vi "891 Software.vi"() -> ()   [LabVIEW 2020]
doc: "This Continuous Measurement sample project is based on the Queued Message Handler template.\n\nThe Event Handling Loop generates messages based on user interface actions.\n\nThe Message Handling Loop processes messages generated by the Event Handling Loop, or by other messages. There are also Acquisition and Logging message handling loop subVIs, and a chart updating loop."
uses:
  2840 Software/controls/Instrument Refs.ctl
  Settings/Settings.ctl
  controls/UI Data.ctl
  controls/UI State.ctl
  controls/UI Sweep.ctl
  support/Message Queue/Enqueue Message (Single).vi
  support/Message Queue/Enqueue Message (Array).vi
  <vilib>/Utility/error.llb/Error Cluster From Error Code.vi
  <vilib>/regexp/Match Regular Expression.xnode
  <vilib>/ErrorRing/Error Ring.xnode
  Acquisition/Acquisition.lvlib
  Logging/Logging.lvlib
  Settings/Settings.lvlib
  support/User Event - Stop/User Event - Stop.lvlib
  support/Message Queue/Message Queue.lvlib
  891 software library/Copy of Copy of BK Precision 891.lvlib
  Settings/Settings Dialog.vi
panel:
  in  "Disconnect":bool
  out "Enable Sweep New Value":bool
  out "NewVal":enum32{"BIN", "SWEEP"}(ring)
  out "Tab Ref":refnum<vi>
  out "OldVal":dbl
  out "CtlRef":refnum<vi>
  out "New High Limit Val":dbl
  out "High Limit Ref":refnum<vi>
  out "Low Limit Ref":refnum<vi>
  out "New Low Limit Val":dbl
  out "BIN REF":refnum<vi>
  out "New BIN State":bool
  in  "BIN Read In":T1
  in  "?":T2
  out "Function":string
  out "Secondary":string
  out "Primary":string
  out "Color Box":u32(colorbox)=11347
  in  "Frequency":dbl=1000.0 format="%#_4p"
  in  "Level":u8(ring) items=["0.5Vrms", "1Vrms"]
  in  "Range":u16(ring)=1 items=["Hold", "Auto"]
  in  "Speed":u16(ring)=1 items=["Slow"=1, "Fast"=2]
  in  "Function":u16(ring) items=["Cs-Q", "Cs-D", "Cs-R", "Cp-Q", "Cp-D", "Cp-R", "Cp-G", "Ls-Q", "Ls-D", "Ls-R", "Lp-Q", "Lp-D", "Lp-R", "Lp-G", "Z-th", "Y-th", "R-X", "G-B", "DCR"]
  in  "Tab Control":enum32{"BIN", "SWEEP"}(tab)
  in  "High Limit":T3={"BIN 1"=1.0, "BIN 2"=1.0, "BIN 3"=1.0, "BIN 4"=1.0, "BIN 5"=1.0, "BIN 6"=1.0, "BIN 7"=1.0, "BIN 8"=1.0, "BIN 9"=1.0, "SEC"=1.0} {"SEC" min=1.0 step=100.0 format="%#_6p"; "BIN 9" min=1.0 step=100.0 format="%#_6p"; "BIN 8" min=1.0 step=100.0 format="%#_6p"; "BIN 7" min=1.0 step=100.0 format="%#_6p"; "BIN 6" min=1.0 step=100.0 format="%#_6p"; "BIN 5" min=1.0 step=100.0 format="%#_6p"; "BIN 4" min=1.0 step=100.0 format="%#_6p"; "BIN 3" min=1.0 step=100.0 format="%#_6p"; "BIN 2" min=1.0 step=100.0 format="%#_6p"; "BIN 1" min=1.0 step=100.0 format="%#_6p"}
  in  "Low Limit":T3 {"SEC" step=100.0 format="%#_6p"; "BIN 9" step=100.0 format="%#_6p"; "BIN 8" step=100.0 format="%#_6p"; "BIN 7" step=100.0 format="%#_6p"; "BIN 6" step=100.0 format="%#_6p"; "BIN 5" step=100.0 format="%#_6p"; "BIN 4" step=100.0 format="%#_6p"; "BIN 3" step=100.0 format="%#_6p"; "BIN 2" step=100.0 format="%#_6p"; "BIN 1" step=100.0 format="%#_6p"}
  in  "BIN State Read":bool
  in  "Clear Count":bool=TRUE
  in  "Comparator Swap":bool
  in  "Trigger":bool=TRUE
  in  "Count State":bool
  in  "Beeper Mode":u16(ring) items=["Off", "Beep when Pass", "Beep when Failed"]
  in  "Comparator Mode":u16(ring) items=["Tolerance", "Absolute"]
  in  "Bin Display Mode":u16(ring) items=["BIN", "Table", "Histogram"]
  in  "Nominal Value (0.0)":dbl step=100.0
  in  "BIN No.":T4
  out "BIN 1":bool
  out "BIN 2":bool
  out "BIN 3":bool
  out "BIN 4":bool
  out "BIN 5":bool
  out "BIN 6":bool
  out "BIN 7":bool
  out "BIN 8":bool
  out "BIN 9":bool
  out "BIN 10":bool
  out "BIN Result":i32[](array[numeric]) format="%.0p"
  out "Nominal":string
  out "Low Limit Read":dbl[](array[numeric]) format="%#_6p"
  out "High Limit Read":dbl[](array[numeric]) format="%#_6p"
  in  "Sweep Function":u16(ring) items=["Cs-Q", "Cs-D", "Cs-R", "Cp-Q", "Cp-D", "Cp-R", "Cp-G", "Ls-Q", "Ls-D", "Ls-R", "Lp-Q", "Lp-D", "Lp-R", "Lp-G", "Z-th", "Y-th", "R-X", "G-B", "DCR"]
  out "XY Graph":cluster{dbl[], dbl[]}(graph)
  in  "Interpolation":u16(ring) items=["Disable", "Enable"]
  in  "Sweep Display Mode":u16(ring) items=["Graph", "Table"]
  in  "Autoscale Limit":bool=TRUE
  in  "Sweep Low Limit":dbl format="%#.3f"
  in  "Sweep High Limit":dbl format="%#.3f"
  in  "Start Frequency":dbl=20.0 min=20.0 max=300000.0 format="%.1f"
  in  "Stop Frequency":dbl=1000.0 min=20.0 max=300000.0 format="%.1f"
  in  "Sweep Points":i32(ring) items=["300 ", "150", "60", "30"]
  in  "Autoscale Frequency":bool=TRUE
  in  "Sweep Parameter":u16(ring) items=["Primary", "Secondary"]
  in  "Sweep Mode":u16(ring) items=["Linear", "Logarithmic"]
  in  "Enable Sweep":bool
  in  "Log File Path":path
  in  "Connect":bool=TRUE
  in  "Reset (True)":bool=TRUE
  in  "Select LCR":refnum<visa-resource-name>="COM12"
  in  "Settings":bool
  in  "Start":bool
  in  "Stop":bool
  in  "Disconnect":bool
  out "FW Ver.":string="/ 1.68 / 4.02B\r\n"
  out "SN":string="BK001, 3."
  out "Model":string="891"
  out "IDN":string="B&K Precision ,891,BK001, 3.02/ 1.68 / 4.02B\r\n"
  out "Status":string="Exit"
  # "Measurement"
  # "Signal Configuration"
  # "1"
  # "2"
  # "3"
  # "4"
  # "5"
  # "6"
  # "7"
  # "8"
  # "9"
  # "SEC"
  # "OUT"
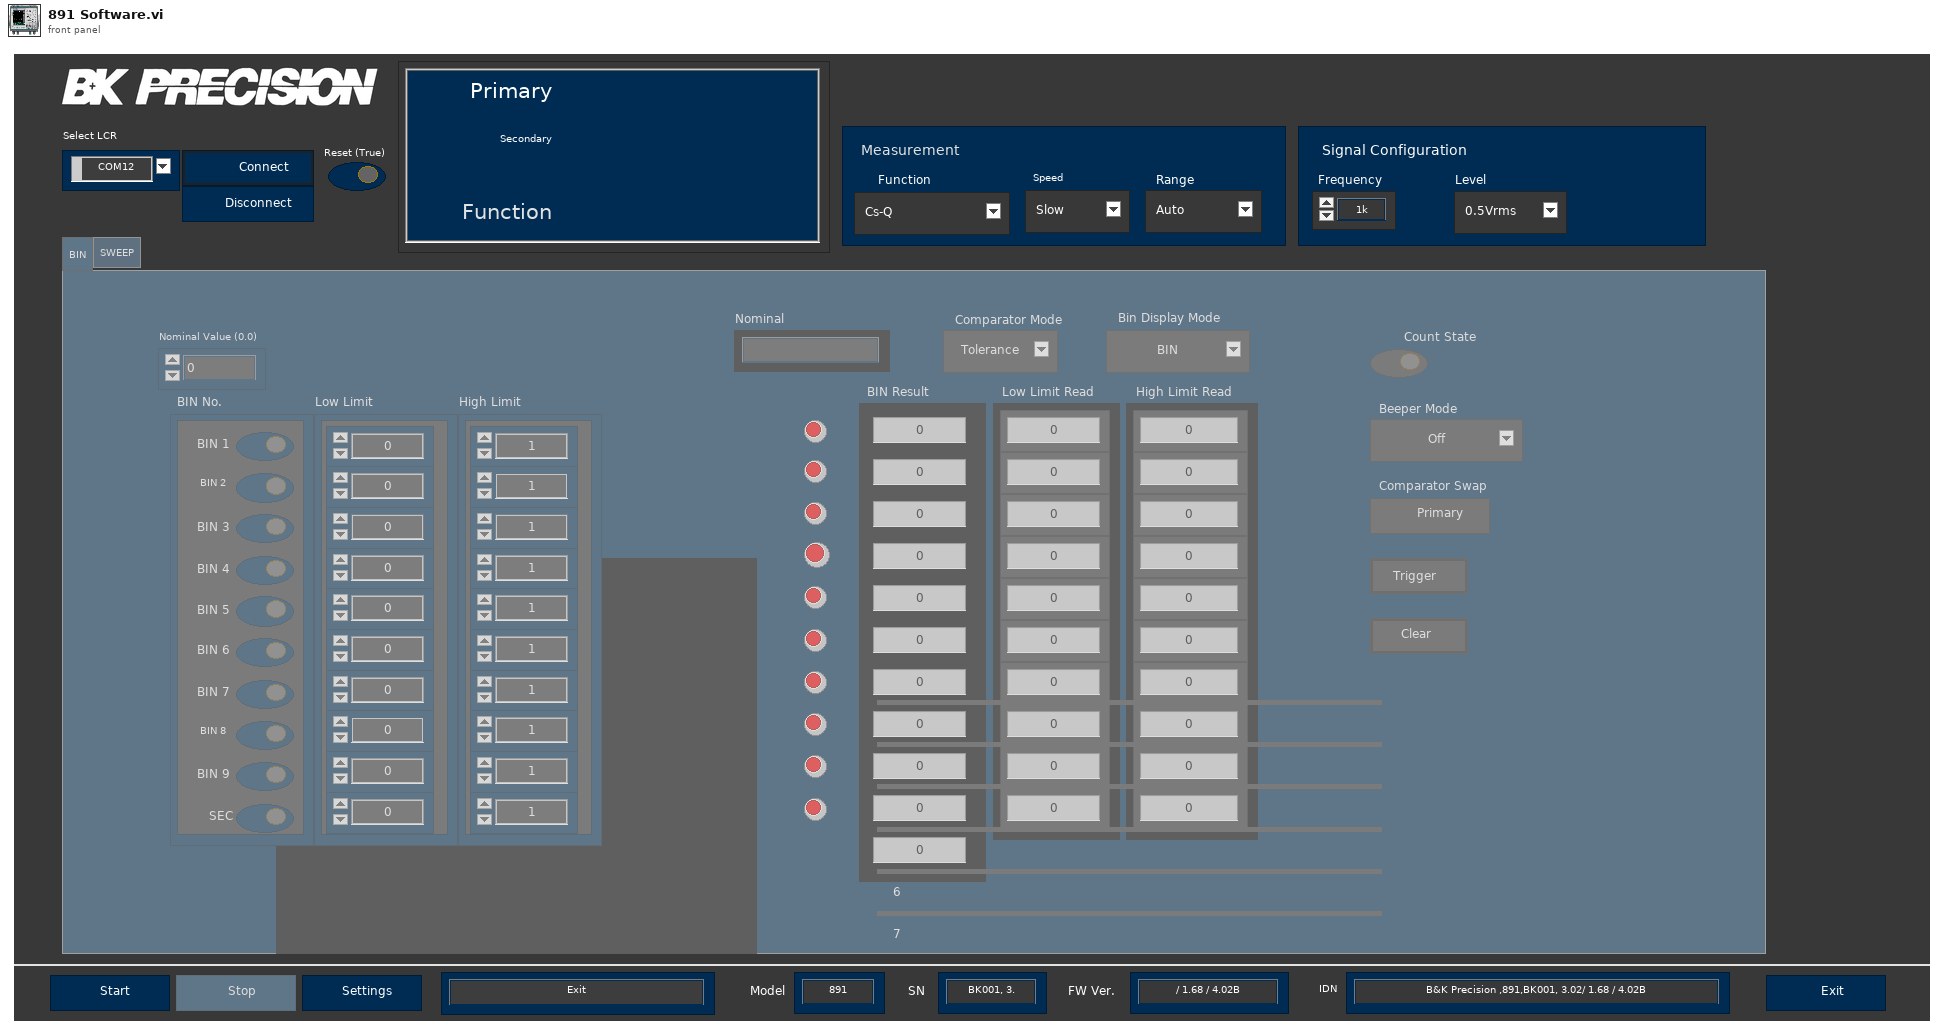
[diagram p1: front panel]
types:
  T1 = cluster{"Low Limit Read":dbl[], "High Limit Read":dbl[], "BIN Count Array":i32[], "Nominal":string}
  T2 = typedef "Instrument Refs.ctl" = cluster{"Function":refnum<vi>, "BIN 1":refnum<vi>, "BIN 2":refnum<vi>, "BIN 3":refnum<vi>, "BIN 4":refnum<vi>, "BIN 5":refnum<vi>, "BIN 6":refnum<vi>, "BIN 7":refnum<vi>, "BIN 8":refnum<vi>, "BIN 9":refnum<vi>, "BIN 10":refnum<vi>}
  T3 = cluster{"BIN 1":dbl, "BIN 2":dbl, "BIN 3":dbl, "BIN 4":dbl, "BIN 5":dbl, "BIN 6":dbl, "BIN 7":dbl, "BIN 8":dbl, "BIN 9":dbl, "SEC":dbl}
  T4 = cluster{"BIN 1":bool, "BIN 2":bool, "BIN 3":bool, "BIN 4":bool, "BIN 5":bool, "BIN 6":bool, "BIN 7":bool, "BIN 8":bool, "BIN 9":bool, "SEC":bool}
  T5 = typedef "UI Sweep.ctl" = cluster{"Function Ref":refnum<vi>, "Speed Ref":refnum<vi>, "Range Ref":refnum<vi>, "Comparator Ref":refnum<vi>, "BIN Display Ref":refnum<vi>, "Enable Count Ref":refnum<vi>, "Beeper Ref":refnum<vi>, "BIN NO. Ref":refnum<vi>, "Low Limit Ref":refnum<vi>, "High Limit Ref":refnum<vi>, "Nominal Value Ref":refnum<vi>, "Enable Sweep":refnum<vi>, "Sweep Mode Ref":refnum<vi>, "Sweep Display Mode Ref":refnum<vi>, "Sweep Parameter Ref":refnum<vi>, "Interporlation Ref":refnum<vi>, "Sweep Step Ref":refnum<vi>, "Autoscale Sweep":refnum<vi>, "Start Freq Ref":refnum<vi>, "Stop Freq Ref":refnum<vi>, "Autoscale Frequency":refnum<vi>, "Sweep Low Limit Ref":refnum<vi>, "Sweep High Limit Ref":refnum<vi>, "Freq Ref":refnum<vi>, "Level Ref":refnum<vi>, "TabCtl Refnum":refnum<vi>}
  T6 = typedef "UI State.ctl" = enum16{"Idle", "Acquiring and Logging", "Waiting for Exit", "Waiting for Exit (Acq Stopped)", "Waiting for Exit (Log Stopped)", "Waiting for Stop", "Waiting for Stop (Acq Stopped)", "Waiting for Stop (Log Stopped)", "Waiting for Sweep(Sweep Complete)"}
  T7 = typedef "UI Data.ctl" = cluster{"Start Ref":refnum<vi>, "Stop Ref":refnum<vi>, "Settings Ref":refnum<vi>, "Exit Ref":refnum<vi>, "Status Ref":refnum<vi>, "Function Ref":refnum<vi>, "Range Ref":refnum<vi>, "Speed Ref":refnum<vi>, "Level Ref":refnum<vi>, "Freq Refnum":refnum<vi>, "Sweep ":refnum<vi>, "Autoscale Sweep":refnum<vi>, "Autoscale Frequency":refnum<vi>, "TabCtl Refnum":refnum<vi>}
  T8 = typedef "Settings.lvlib/Settings.ctl" = cluster{"VISA resource name":refnum<visa-resource-name>, "Logging Configuration":cluster{"Byte Stream File Refnum":refnum<file>, "File Path":path, "String":string}, "Comparator Mode":u16, "BIN State":bool, "Start Ref":refnum<vi>, "Stop Ref":refnum<vi>}
  T9 = typedef "Message Queue.lvlib/All Message Queues.ctl" = cluster{"UI":refnum<queue>, "Acquisition":refnum<queue>, "Logging":refnum<queue>}
  T10 = enum8{"Enabled", "Disabled", "Disabled and Grayed Out"}
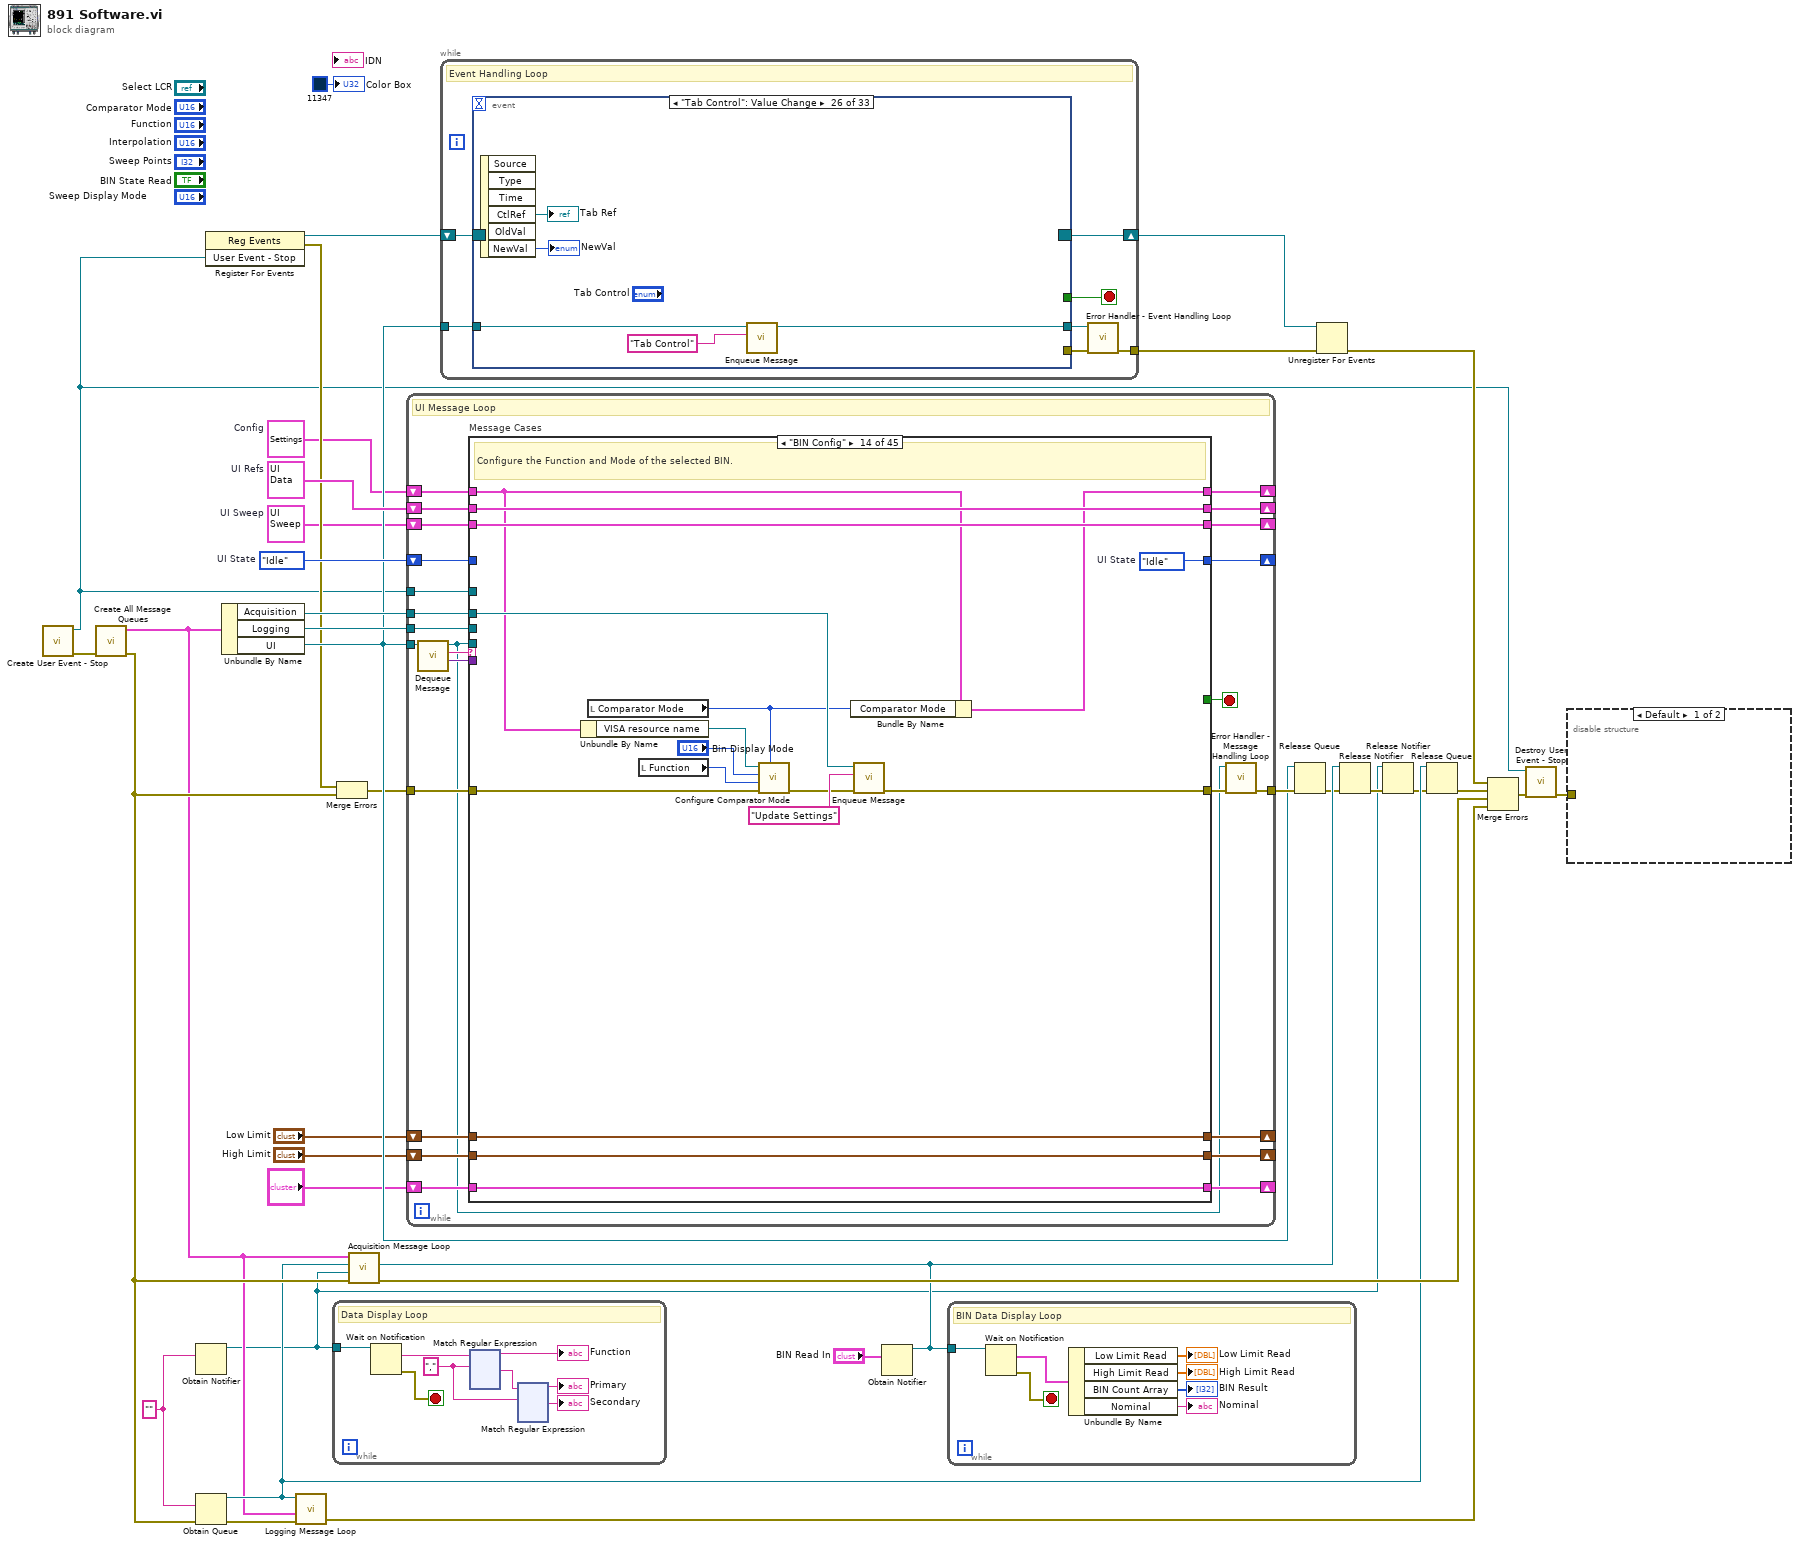
[diagram p0: block diagram]
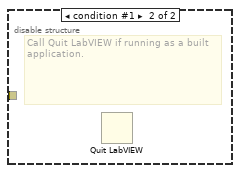
[diagram p2: hidden frame]
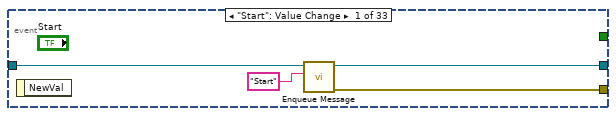
[diagram p3: hidden frame]
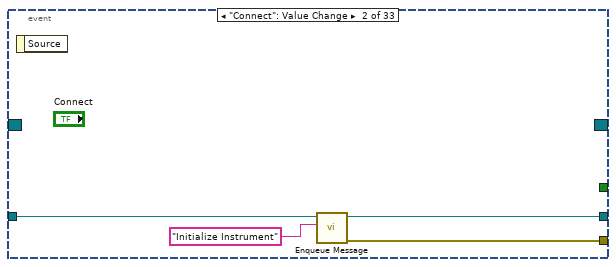
[diagram p4: hidden frame]
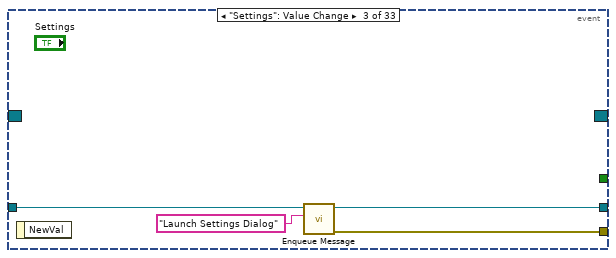
[diagram p5: hidden frame]
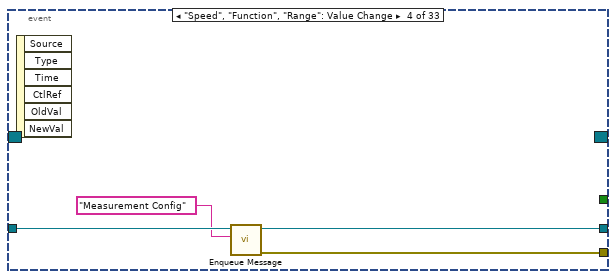
[diagram p6: hidden frame]
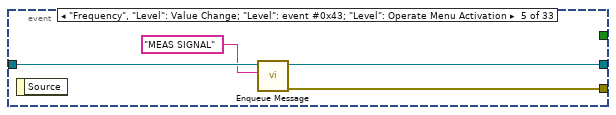
[diagram p7: hidden frame]
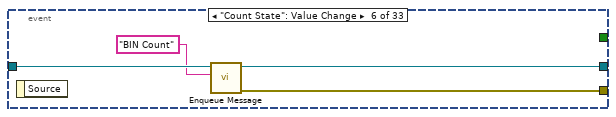
[diagram p8: hidden frame]
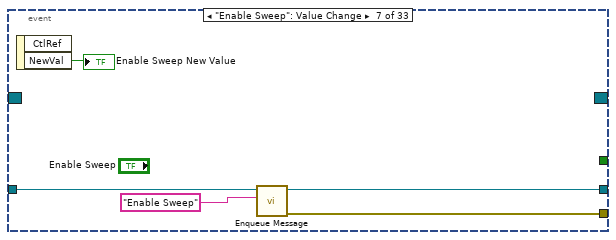
[diagram p9: hidden frame]
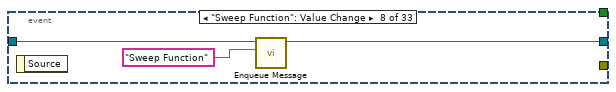
[diagram p10: hidden frame]
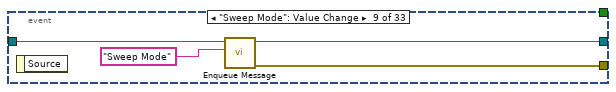
[diagram p11: hidden frame]
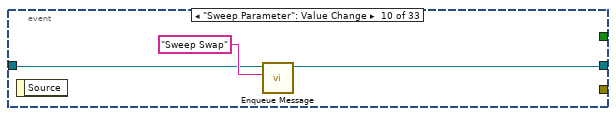
[diagram p12: hidden frame]
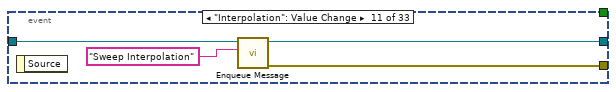
[diagram p13: hidden frame]
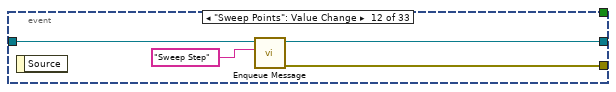
[diagram p14: hidden frame]
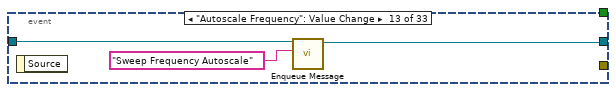
[diagram p15: hidden frame]
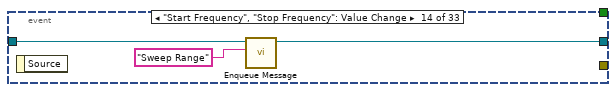
[diagram p16: hidden frame]
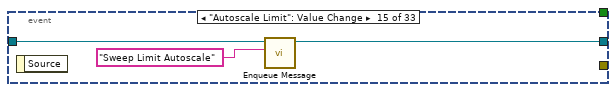
[diagram p17: hidden frame]
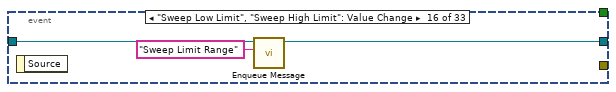
[diagram p18: hidden frame]
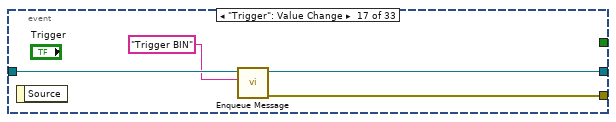
[diagram p19: hidden frame]
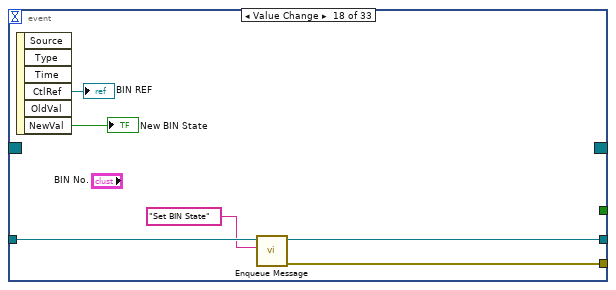
[diagram p20: hidden frame]
diagram:
  w18 = T5 {"Function Ref"=refnum, "Speed Ref"=refnum, "Range Ref"=refnum, "Comparator Ref"=refnum, "BIN Display Ref"=refnum, "Enable Count Ref"=refnum, "Beeper Ref"=refnum, "BIN NO. Ref"=refnum, "Low Limit Ref"=refnum, "High Limit Ref"=refnum, "Nominal Value Ref"=refnum, "Enable Sweep"=refnum, "Sweep Mode Ref"=refnum, "Sweep Display Mode Ref"=refnum, "Sweep Parameter Ref"=refnum, "Interporlation Ref"=refnum, "Sweep Step Ref"=refnum, "Autoscale Sweep"=refnum, "Start Freq Ref"=refnum, "Stop Freq Ref"=refnum, "Autoscale Frequency"=refnum, "Sweep Low Limit Ref"=refnum, "Sweep High Limit Ref"=refnum, "Freq Ref"=refnum, "Level Ref"=refnum, "TabCtl Refnum"=refnum}  # UI Sweep
  w20 = ""
  w27 = UI_State."Idle"  # UI State
  w30 = T7 {"Start Ref"=refnum, "Stop Ref"=refnum, "Settings Ref"=refnum, "Exit Ref"=refnum, "Status Ref"=refnum, "Function Ref"=refnum, "Range Ref"=refnum, "Speed Ref"=refnum, "Level Ref"=refnum, "Freq Refnum"=refnum, "Sweep "=refnum, "Autoscale Sweep"=refnum, "Autoscale Frequency"=refnum, "TabCtl Refnum"=refnum}  # UI Refs
  w17 = T8 {"VISA resource name"="COM1", "Logging Configuration"={"Byte Stream File Refnum"=refnum, "File Path"=path "", "String"=""}, "Comparator Mode"=1, "BIN State"=FALSE, "Start Ref"=refnum, "Stop Ref"=refnum}  # Config
  n1 = call "Create User Event - Stop.vi"() -> ("error out"=w33:errorcluster, "User Event - Stop"=w4:refnum<user-event>)  [unwired: 10 in]
  n2 = call "Create All Message Queues.vi"("error in (no error)"=w33) -> ("error out"=w15:errorcluster, "Message Queues out"=w9:T9)  [unwired: 9 in]
  n3 = Obtain Notifier(notification data type=w20) -> (notifier out=w5:refnum<notifier>)  [unwired: 3 in, 2 out]
  n4 = Obtain Queue(element data type=w20, error in (no error)=w15) -> (queue out=w10:refnum<queue>, error out=w16:errorcluster)  [unwired: 3 in, 1 out]
  n5 = register-events(w4) -> (reference out=w23:refnum<event-registration>, error out=w21:errorcluster)  [unwired: 2 in]
  n6 = Unbundle By Name(w9) -> ("Acquisition"=w29:refnum<queue>, "Logging"=w28:refnum<queue>, "UI"=w25:refnum<queue>)
  n7 = call "Logging Message Loop.vi"("error in (no error)"=w16, "Message Queues"=w9, "Data Queue"=w10) -> ("error out"=w32:errorcluster)  [unwired: 8 in]
  n8 = while "Data Display Loop" {
    tunnel: w5 -> [w44]
    stop <- w43 stop-if-true
    w39 = "," ("regular expression")
    # "Data Display Loop"
    n9 = Wait on Notification(notifier=w44) -> (notification=w40:string, error out=w43:errorcluster)  [unwired: 3 in, 2 out]
    n10 = xnode "Match Regular Expression"("input string"=w40, "regular expression"=w39) -> ("before match"=→"Function":string, "after match"=w38:string)  [unwired: 4 in, 3 out]
    n11 = xnode "Match Regular Expression"("input string"=w38, "regular expression"=w39) -> ("before match"=→"Primary":string, "after match"=→"Secondary":string)  [unwired: 4 in, 3 out]
  }
  n12 = Merge Errors(w21, w15) -> (w22:errorcluster)
  n13 = while {
    tunnel: w25 -> [w293]
    tunnel: w4 -> [w296]
    shift-right: [w292] -> _
    shift-left: w17 -> [w278]
    shift-right: [w290] -> _
    shift-left: w30 -> [w291]
    tunnel: w29 -> [w289]
    tunnel: w28 -> [w288]
    shift-right: [w284] -> _
    shift-left: w27 -> [w285]
    tunnel: w22 -> [w283]
    tunnel: [w287] -> w36
    shift-right: [w281] -> _
    shift-left: w18 -> [w282]
    shift-right: [w279] -> _
    shift-left: "?" -> [w280]
    shift-right: [w274] -> _
    shift-left: "High Limit" -> [w277]
    shift-right: [w275] -> _
    shift-left: "Low Limit" -> [w276]
    stop <- w297 stop-if-true
    # "UI Message Loop"
    n14 = call "Dequeue Message.vi"("Message Queue"=w293) -> ("Message Data"=w294:variant, "Message"=w295:string, "dup Message Queue"=w273:refnum<queue>)  [unwired: 7 in, 1 out]
    n15 = case "Message Cases" shown="\"BIN Config\"" w295 {
      selector: w295 -> [_ _ _ _ _ _ _ _ _ _ _ _ _ _ _ _ _ _ _ _ _ _ _ _ _ _ _ _ _ _ _ _ _ _ _ _ _ _ _ _ _ _ _ _ w1651]
      tunnel: w273 -> [w306 _ _ w389 _ w431 _ _ _ _ _ _ _ _ _ _ _ _ _ w1051 _ _ _ _ _ _ _ _ _ _ w1296 w1333 w1380 _ w1428 w1465 w1496 _ _ w1543 w1579 _ _ _ _]
      tunnel: w283 -> [w309 w322 w376 w412 w425 w433 w461 w491 w504 w526 w665 w812 w945 w970 w985 w995 w1019 w1029 w1047 w1058 w1147 w1163 w1175 w1195 w1210 w1224 w1245 w1252 w1268 w1282 w1298 w1363 w1398 w1418 w1429 w1466 w1498 w1521 w1529 w1542 w1570 w1597 w1623 w1641 _]
      tunnel: [w313 w322 w376 w390 w426 w450 w460 w490 w503 w524 w662 w809 w944 w966 w984 w990 w1016 w1025 w1037 w1061 w1146 w1162 w1173 w1194 w1209 w1223 w1245 w1251 w1267 w1281 w1294 w1336 w1382 w1403 w1426 w1463 w1492 w1522 w1527 w1541 w1571 w1594 w1620 w1641 w1650] -> w286
      tunnel: [_ _ _ _ _ _ _ _ _ _ _ _ _ _ _ _ _ _ _ _ _ _ _ _ _ _ _ _ _ _ _ _ _ _ _ _ _ _ _ _ _ _ TRUE _ _] -> w297
      tunnel: w294 -> [_ _ _ _ w424 _ _ _ _ _ _ _ _ _ _ _ _ _ _ _ _ _ _ _ _ _ _ _ _ _ _ _ _ _ _ _ _ _ w1532 _ _ w1602 w1632 _ _]
      tunnel: w296 -> [_ _ _ _ _ _ _ _ _ _ _ _ _ _ _ _ _ _ _ _ _ _ _ _ _ _ _ _ _ _ _ _ _ _ _ _ _ _ _ _ _ _ w1628 _ _]
      tunnel: [w302 w338 w375 w397 w416 w448 w457 w486 w499 w523 w664 w811 w940 w964 w980 w998 w1014 w1031 w1042 w1059 w1143 w1159 w1176 w1193 w1207 w1222 w1236 w1250 w1270 w1278 w1292 w1356 w1378 w1401 w1423 w1458 w1491 w1512 w1525 w1537 w1573 w1588 w1626 w1639 w1647] -> w292
      tunnel: w291 -> [w310 w348 w380 w403 w420 w454 w466 w496 w508 w533 w669 w816 w950 w977 w988 w1002 w1022 w1035 w1049 w1062 w1155 w1170 w1183 w1198 w1217 w1230 w1244 w1258 w1274 w1289 w1301 w1360 w1396 w1417 w1431 w1457 w1494 w1520 w1534 w1545 w1583 w1605 w1635 w1644 w1653]
      tunnel: [w310 w346 w380 w403 w420 w454 w466 w496 w508 w533 w669 w816 w950 w977 w988 w1002 w1022 w1035 w1049 w1062 w1155 w1170 w1183 w1198 w1217 w1230 w1244 w1258 w1274 w1289 w1301 w1360 w1396 w1417 w1431 w1457 w1494 w1520 w1534 w1545 w1583 w1605 w1635 w1644 w1653] -> w290
      tunnel: w289 -> [_ _ _ _ _ w451 _ _ _ _ _ _ _ w968 _ w989 _ w1027 w1036 w1052 _ _ _ _ _ _ _ _ _ _ _ w1337 _ _ _ _ _ w1519 _ _ w1581 w1585 w1624 _ _]
      tunnel: w288 -> [_ _ _ _ _ _ _ _ _ _ _ _ _ _ _ _ _ _ _ _ _ _ _ _ _ _ _ _ _ _ _ _ w1386 w1407 _ _ _ w1518 _ _ w1576 w1586 w1625 _ _]
      tunnel: w285 -> [_ _ _ w413 w419 w453 w455 w494 w502 w531 w645 w796 w943 _ w982 w1000 w1017 w1033 w1045 w1055 w1145 w1167 w1181 w1191 w1205 w1227 w1241 w1255 w1272 w1279 _ w1339 _ w1405 w1430 w1467 w1493 w1517 w1531 w1544 w1580 _ _ w1643 w1652]
      tunnel: [UI_State."Idle" ("UI State") UI_State."Idle" ("UI State") w379 w413 w419 w453 w455 w494 w502 w531 w645 w796 w943 w976 w982 w1000 w1017 w1033 w1045 w1055 w1145 w1167 w1181 w1191 w1205 w1227 w1241 w1255 w1272 w1279 w1300 w1339 UI_State."Acquiring and Logging" ("UI State") w1406 w1427 w1464 w1493 w1517 w1531 w1540 w1580 UI_State."Idle" ("UI State") UI_State."Idle" ("UI State") w1643 w1652] -> w284
      tunnel: [w300 w336 w377 w398 w418 w452 w465 w495 w501 w532 w668 w815 w949 w975 w987 w1001 w1021 w1034 w1048 w1056 w1144 w1169 w1182 w1187 w1216 w1229 w1243 w1257 w1273 w1280 w1299 w1355 w1384 w1404 w1425 w1462 w1490 w1516 w1528 w1539 w1582 w1592 w1616 w1642 w1649] -> w281
      tunnel: w282 -> [w301 w336 w378 w398 w418 w452 w465 w495 w501 w532 w668 w815 w949 w975 w987 w1001 w1021 w1034 w1048 w1056 w1144 w1169 w1182 w1187 w1216 w1229 w1243 w1257 w1273 w1280 w1299 w1355 w1384 w1404 w1425 w1462 w1490 w1516 w1528 w1539 w1582 w1592 w1616 w1642 w1649]
      tunnel: w280 -> [w304 w334 w353 w388 w417 w434 w464 w487 w500 w530 w667 w814 w948 w974 w981 w999 w1015 w1032 w1043 w1060 w1154 w1168 w1180 w1197 w1215 w1228 w1242 w1256 w1271 w1288 w1293 w1357 w1379 w1402 w1424 w1461 w1489 w1507 w1526 w1538 w1574 w1598 w1627 w1640 w1648]
      tunnel: [w304 w333 w353 w388 w417 w434 w464 w487 w500 w530 w667 w814 w948 w974 w981 w999 w1015 w1032 w1043 w1060 w1154 w1168 w1180 w1197 w1215 w1228 w1242 w1256 w1271 w1288 w1293 w1357 w1379 w1402 w1424 w1461 w1489 w1507 w1526 w1538 w1574 w1598 w1627 w1640 w1648] -> w279
      tunnel: w278 -> [w303 w321 w375 w387 w416 w448 w457 w486 w499 w523 w664 w811 w940 w965 w980 w998 w1014 w1031 w1042 w1059 w1143 w1159 w1176 w1193 w1207 w1222 w1236 w1250 w1270 w1278 w1292 w1356 w1378 w1401 w1423 w1458 w1488 w1506 w1525 w1537 w1573 w1588 w1626 w1639 w1647]
      tunnel: w277 -> [w298 w317 w349 w382 w414 w427 w462 w484 w497 w509 w648 w793 w946 w961 w978 w992 w1012 w1023 w1040 w1053 w1136 w1156 w1171 w1188 w1203 w1218 w1233 w1246 w1261 w1275 w1290 w1329 w1376 w1399 w1421 w1459 w1486 w1504 w1523 w1535 w1567 w1590 w1614 w1637 w1645]
      tunnel: w276 -> [w299 w318 w350 w383 w415 w428 w463 w485 w498 w510 w647 w794 w947 w962 w979 w993 w1013 w1024 w1041 w1054 w1137 w1157 w1172 w1189 w1204 w1219 w1234 w1247 w1262 w1276 w1291 w1330 w1377 w1400 w1422 w1460 w1487 w1505 w1524 w1536 w1568 w1591 w1615 w1638 w1646]
      tunnel: [w299 w318 w350 w383 w415 w428 w463 w485 w498 w510 w646 w794 w947 w962 w979 w993 w1013 w1024 w1041 w1054 w1137 w1157 w1172 w1189 w1204 w1219 w1234 w1247 w1262 w1276 w1291 w1330 w1377 w1400 w1422 w1460 w1487 w1505 w1524 w1536 w1568 w1591 w1615 w1638 w1646] -> w275
      tunnel: [w298 w317 w349 w382 w414 w427 w462 w484 w497 w509 w648 w792 w946 w961 w978 w992 w1012 w1023 w1040 w1053 w1136 w1156 w1171 w1188 w1203 w1218 w1233 w1246 w1261 w1275 w1290 w1329 w1376 w1399 w1421 w1459 w1486 w1504 w1523 w1535 w1567 w1590 w1614 w1637 w1645] -> w274
      frame "Initialize" {
        # "Initialize - Get configuration settings, then message the UI to initialize, and broadcast the settings to the other message loops."
        n16 = call-poly "Enqueue Message.vi"("error in (no error)"=w309, "Message Array"=string[] ["Init UI Refs", "Set Controls Ref", "Broadcast Settings"], "Message Queue"=w306) -> ("error out"=w314:errorcluster, "dup Message Queue"=w305:refnum<queue>)  [unwired: 7 in]
        n17 = call-poly "Enqueue Message.vi"("error in (no error)"=w314, "Message Data"="Ready..." ("Ready..."), "Message"="Update Status", "Message Queue"=w305) -> ("error out"=w313:errorcluster)  [unwired: 6 in, 1 out]
        n18 = call "Load Settings from XML.vi"("Settings in"=w303) -> ("Settings out"=w302:T8)  [unwired: 9 in, 1 out]
        n19 = call "Load Default UI Settings.vi"("UI Sweep"=w301) -> ("UI Sweep OUT"=w300:T5)  [unwired: 9 in, 1 out]
      }
      frame "Init UI Refs" {
        w319 = T10."Disabled and Grayed Out" ("Disabled")
        w320 = T10."Disabled and Grayed Out" ("Disabled")
        # "Init UI Refs - Store control references for UI controls.  Also enable/disable controls appropriately."
        n20 = control-ref of="BIN 1"() -> (w327:refnum<vi>)
        n21 = control-ref of="BIN 2"() -> (w328:refnum<vi>)
        n22 = control-ref of="BIN 3"() -> (w329:refnum<vi>)
        n23 = control-ref of="BIN 4"() -> (w330:refnum<vi>)
        n24 = control-ref of="BIN 5"() -> (w331:refnum<vi>)
        n25 = control-ref of="BIN 6"() -> (w332:refnum<vi>)
        n26 = control-ref of="BIN 7"() -> (w326:refnum<vi>)
        n27 = control-ref of="BIN 8"() -> (w325:refnum<vi>)
        n28 = control-ref of="BIN 9"() -> (w324:refnum<vi>)
        n29 = control-ref of="BIN 10"() -> (w323:refnum<vi>)
        n30 = control-ref of="Start"() -> (w316:refnum<vi>)
        n31 = control-ref of="Stop"() -> (w315:refnum<vi>)
        n32 = control-ref of="Settings"() -> (w341:refnum<vi>)
        n33 = control-ref of="Disconnect"() -> (w340:refnum<vi>)
        n34 = control-ref of="Tab Control"() -> (w335:refnum<vi>)
        n35 = property on="Start Frequency" class="DigNum (strict)"("DisabledEnum"=w320) -> ()  [unwired: 2 in, 2 out]
        n36 = property on="Stop Frequency" class="DigNum (strict)"("DisabledEnum"=w320) -> ()  [unwired: 2 in, 2 out]
        n37 = control-ref of="Status"() -> (w347:refnum<vi>)
        n38 = Build Array(w316, w341, w340) -> (w344:refnum<vi>[])
        n39 = Bundle By Name(cluster=w334, "BIN 1"=w327, "BIN 2"=w328, "BIN 3"=w329, "BIN 4"=w330, "BIN 5"=w331, "BIN 6"=w332, "BIN 7"=w326, "BIN 8"=w325, "BIN 9"=w324, "BIN 10"=w323) -> (w333:T2)
        n40 = call "Set Enable State on Multiple Controls.vi"("Enable?"=TRUE, "Controls"=w344) -> ()  [unwired: 10 in]
        n41 = Bundle By Name(cluster=w348, "Start Ref"=w316, "Stop Ref"=w315, "Settings Ref"=w341, "Exit Ref"=w340, "Status Ref"=w347, "TabCtl Refnum"=w335) -> (w346:T7)
        n42 = property on="Sweep Low Limit" class="DigNum (strict)"("DisabledEnum"=w319) -> ()  [unwired: 2 in, 2 out]
        n43 = property on="Sweep High Limit" class="DigNum (strict)"("DisabledEnum"=w319) -> ()  [unwired: 2 in, 2 out]
        n44 = Bundle By Name(cluster=w321, "Logging Configuration.File Path"="Log File Path") -> (w338:T8)
        n45 = Build Array(w315, w335) -> (w343:refnum<vi>[])
        n46 = call "Set Enable State on Multiple Controls.vi"("Enable?"=FALSE, "Controls"=w343) -> ()  [unwired: 10 in]
      }
      frame "Set Controls Ref" {
        w379 = UI_State."Idle"  # UI State
        # "BIN Refs"
        # "Sweep Config"
        # "Signal Config Ref"
        # "Measurement Ref"
        n47 = control-ref of="Count State"() -> (w370:refnum<vi>)
        n48 = control-ref of="Enable Sweep"() -> (w369:refnum<vi>)
        n49 = control-ref of="Autoscale Limit"() -> (w360:refnum<vi>)
        n50 = control-ref of="Autoscale Frequency"() -> (w357:refnum<vi>)
        n51 = control-ref of="BIN No."() -> (w367:refnum<vi>)
        n52 = control-ref of="Nominal Value (0.0)"() -> (w366:refnum<vi>)
        n53 = control-ref of="Start Frequency"() -> (w359:refnum<vi>)
        n54 = control-ref of="Stop Frequency"() -> (w358:refnum<vi>)
        n55 = control-ref of="Sweep Low Limit"() -> (w356:refnum<vi>)
        n56 = control-ref of="Sweep High Limit"() -> (w355:refnum<vi>)
        n57 = control-ref of="Frequency"() -> (w365:refnum<vi>)
        n58 = control-ref of="Function"() -> (w351:refnum<vi>)
        n59 = control-ref of="Speed"() -> (w374:refnum<vi>)
        n60 = control-ref of="Range"() -> (w373:refnum<vi>)
        n61 = control-ref of="Comparator Mode"() -> (w372:refnum<vi>)
        n62 = control-ref of="Bin Display Mode"() -> (w371:refnum<vi>)
        n63 = control-ref of="Beeper Mode"() -> (w368:refnum<vi>)
        n64 = control-ref of="Sweep Mode"() -> (w364:refnum<vi>)
        n65 = control-ref of="Sweep Display Mode"() -> (w352:refnum<vi>)
        n66 = control-ref of="Sweep Parameter"() -> (w363:refnum<vi>)
        n67 = control-ref of="Interpolation"() -> (w362:refnum<vi>)
        n68 = control-ref of="Sweep Points"() -> (w361:refnum<vi>)
        n69 = control-ref of="Level"() -> (w354:refnum<vi>)
        n70 = Bundle By Name(cluster=w378, "Function Ref"=w351, "Speed Ref"=w374, "Range Ref"=w373, "Comparator Ref"=w372, "BIN Display Ref"=w371, "Enable Count Ref"=w370, "Beeper Ref"=w368, "BIN NO. Ref"=w367, "Nominal Value Ref"=w366, "Enable Sweep"=w369, "Sweep Mode Ref"=w364, "Sweep Display Mode Ref"=w352, "Sweep Parameter Ref"=w363, "Interporlation Ref"=w362, "Sweep Step Ref"=w361, "Autoscale Sweep"=w360, "Start Freq Ref"=w359, "Stop Freq Ref"=w358, "Autoscale Frequency"=w357, "Sweep Low Limit Ref"=w356, "Sweep High Limit Ref"=w355, "Freq Ref"=w365, "Level Ref"=w354) -> (w377:T5)
      }
      frame "Initialize Instrument" {
        # "Initialize instrument. \"Open session, gets identification string, and resets the instrument\""
        n71 = local read "Select LCR"() -> (w395:refnum<visa-resource-name>)
        n72 = call "Initialize.vi"("Reset (True)"="Reset (True)", "ID Query (True)"=TRUE, "error in (no error)"=w412, "VISA resource name"=w395) -> ("error out"=w384:errorcluster, "*IDN?"=w393:string)  [unwired: 5 in, 1 out]
        n73 = Bundle By Name(cluster=w387, "VISA resource name"=w395) -> (w397:T8)
        n74 = String Subset(string=w393, offset (0)=15, length (rest)=3) -> (substring=→"Model":string)
        n75 = property on="Connect" class="Bool (strict)"("DisabledEnum"=T10."Disabled and Grayed Out" ("Disabled")) -> ()  [unwired: 2 in, 2 out]
        n76 = local write "IDN"(w393) -> ()
        n77 = String Subset(string=w393, offset (0)=19, length (rest)=9) -> (substring=→"SN":string)
        n78 = String Subset(string=w393, offset (0)=30, length (rest)=19) -> (substring=→"FW Ver.":string)
        n79 = call-poly "Enqueue Message.vi"("error in (no error)"=w384, "Message"="Broadcast Settings", "Message Queue"=w389) -> ("error out"=w391:errorcluster)  [unwired: 7 in, 1 out]
        n80 = Unbundle By Name(w403) -> ("TabCtl Refnum"=w400:refnum<vi>)
        n81 = call-poly "Enqueue Message.vi"("error in (no error)"=w391, "Message"="Get MEAS", "Message Queue"=w389) -> ("error out"=w390:errorcluster)  [unwired: 7 in, 1 out]
        n82 = Build Array(w400) -> (w401:refnum<vi>[])
        n83 = Wait (ms)(milliseconds to wait=u32 1500) -> ()  [unwired: 1 out]
        n84 = call "Set Enable State on Multiple Controls.vi"("Enable?"=TRUE, "Controls"=w401) -> ()  [unwired: 10 in]
      }
      frame "Update Status" {
        # "Update Status - Convert the message data to a string to display in the Status indicator."
        n85 = Variant To Data(error in=w425, type="", Variant=w424) -> (data=→"Status":string, error out=w422:errorcluster)
        n86 = Merge Errors(w422) -> (w426:errorcluster)
      }
      frame "Get MEAS" {
        # "Starts data acquisition and sets BIN indicators to false"
        n87 = Unbundle By Name(w434) -> ("BIN 1"=w435:refnum<vi>, "BIN 2"=w447:refnum<vi>, "BIN 3"=w446:refnum<vi>, "BIN 4"=w445:refnum<vi>, "BIN 5"=w440:refnum<vi>, "BIN 6"=w444:refnum<vi>, "BIN 7"=w443:refnum<vi>, "BIN 8"=w442:refnum<vi>, "BIN 9"=w441:refnum<vi>, "BIN 10"=w439:refnum<vi>)
        n88 = call-poly "Enqueue Message.vi"("error in (no error)"=w433, "Message Data"="Acquiring " ("Message"), "Message"="Update Status", "Message Queue"=w431) -> ("error out"=w432:errorcluster)  [unwired: 6 in, 1 out]
        n89 = Build Array(w435, w447, w446, w445, w440, w444, w443, w442, w441, w439) -> (w438:refnum<vi>[])
        n90 = Array Size(array=w438) -> (size(s)=w437:i32)
        n91 = call "Set Enable Value on Multiple Controls.vi"("Boolean"=FALSE, "Controls"=w438, "Numeric"=w437) -> ()  [unwired: 9 in]
        n92 = call-poly "Enqueue Message.vi"("error in (no error)"=w432, "Message"="Start", "Message Queue"=w451) -> ("error out"=w450:errorcluster)  [unwired: 7 in, 1 out]
      }
      frame "Tab Control" {
        # "This fixes issues of commands freezing the instrument if\nthe correct page is not selected."
        # "Set display mode based on selected tab."
        n93 = local read "Tab Ref"() -> (w459:refnum<vi>)
        n94 = Unbundle By Name(w457) -> ("VISA resource name"=w456:refnum<visa-resource-name>)
        n95 = property class="TabCtl (strict)"(reference=w459) -> ("Value"=w458:enum32{"BIN", "SWEEP"})  [unwired: 1 in, 2 out]
        n96 = case shown="\"SWEEP\"" w458 {
          tunnel: w461 -> [w475 w483]
          tunnel: [w474 w482] -> w460
          tunnel: w456 -> [w473 w479]
          frame "BIN", Default {
            n97 = property on="Function" class="Ring (strict)"() -> ("Disabled Items []"=w470:i32[])  [unwired: 2 in, 2 out]
            n98 = Format Into String(format string="%.;:DISP:PAGE %d;" ("Input String"), u16 0 ("input 1")) -> (resulting string=w472:string)  [unwired: 2 in, 1 out]
            n99 = Delete From Array(array=w470, length=18) -> (array with subset deleted=w469:i32[])  [unwired: 1 in, 1 out]
            n100 = call "Write.vi"("error in (no error)"=w475, "Input String"=w472, "VISA resource name"=w473) -> ("error out"=w474:errorcluster)  [unwired: 7 in, 1 out]
            n101 = property on="Function" class="Ring (strict)"("Disabled Items []"=w469) -> ()  [unwired: 2 in, 2 out]
          }
          frame "SWEEP" {
            n102 = Build Array(18) -> (w478:i32[])
            n103 = property on="Function" class="Ring (strict)"("Disabled Items []"=w478) -> ()  [unwired: 2 in, 2 out]
            n104 = Format Into String(format string="%.;:DISP:PAGE %d;" ("Input String"), u16 2 ("input 1")) -> (resulting string=w480:string)  [unwired: 2 in, 1 out]
            n105 = call "Write.vi"("error in (no error)"=w483, "Input String"=w480, "VISA resource name"=w479) -> ("error out"=w482:errorcluster)  [unwired: 7 in, 1 out]
          }
        }
      }
      frame "Measurement Config" {
        # "Sets the Measurement parameters\"Function, Speed, Range\""
        n106 = Unbundle By Name(w486) -> ("VISA resource name"=w488:refnum<visa-resource-name>)
        n107 = local read "Function"() -> (w489:u16)
        n108 = call "Configure Measurement.vi"("Function"=w489, "error in (no error)"=w491, "Speed"="Speed", "Range"="Range", "VISA resource name"=w488) -> ("error out"=w490:errorcluster)  [unwired: 5 in, 1 out]
      }
      frame "MEAS SIGNAL" {
        # "Configure the parameters of the testing signal.\"Frequency and amplitude in vrms\""
        n109 = Unbundle By Name(w499) -> ("VISA resource name"=w507:refnum<visa-resource-name>)
        n110 = call "Configure Measurement Signal.vi"("error in (no error)"=w504, "Signal Level (0:0.5 Vrms)"="Level", "Signal Frequency (1000 Hz)"="Frequency", "VISA resource name"=w507) -> ("error out"=w503:errorcluster)  [unwired: 6 in, 1 out]
      }
      frame "Set BIN State" {
        # "Set BIN state."
        n111 = local read "BIN REF"() -> (w529:refnum<vi>)
        n112 = Unbundle By Name(w523) -> ("VISA resource name"=w522:refnum<visa-resource-name>)
        n113 = local read "Comparator Mode"() -> (w525:u16)
        n114 = property on="Property Node" class="Bool (strict)"(reference=w529) -> ("Label.Text"=w528:string)  [unwired: 1 in, 2 out]
        n115 = local read "New BIN State"() -> (w527:bool)
        n116 = local read "New BIN State"() -> (w511:bool)
        n117 = Unbundle By Name(w530) -> ("BIN 1"=w521:refnum<vi>, "BIN 2"=w520:refnum<vi>, "BIN 3"=w519:refnum<vi>, "BIN 4"=w518:refnum<vi>, "BIN 5"=w517:refnum<vi>, "BIN 6"=w516:refnum<vi>, "BIN 7"=w515:refnum<vi>, "BIN 8"=w514:refnum<vi>, "BIN 9"=w513:refnum<vi>, "BIN 10"=w512:refnum<vi>)
        n118 = case shown="\"BIN 2\"" w528 {
          tunnel: w527 -> [w534 w545 w556 w567 w578 w589 w600 w611 w622 w641 _]
          tunnel: w526 -> [w541 w552 w563 w574 w585 w596 w607 w618 w629 w639 w644]
          tunnel: w525 -> [w540 w551 w562 w573 w584 w595 w606 w617 w628 w638 _]
          tunnel: [w538 w549 w560 w571 w582 w593 w604 w615 w626 w637 w644] -> w524
          tunnel: w522 -> [w537 w548 w559 w570 w581 w592 w603 w614 w625 w636 _]
          tunnel: w521 -> [w535 _ _ _ _ _ _ _ _ _ _]
          tunnel: w520 -> [_ w546 _ _ _ _ _ _ _ _ _]
          tunnel: w519 -> [_ _ w557 _ _ _ _ _ _ _ _]
          tunnel: w518 -> [_ _ _ w568 _ _ _ _ _ _ _]
          tunnel: w517 -> [_ _ _ _ w579 _ _ _ _ _ _]
          tunnel: w516 -> [_ _ _ _ _ w590 _ _ _ _ _]
          tunnel: w515 -> [_ _ _ _ _ _ w601 _ _ _ _]
          tunnel: w514 -> [_ _ _ _ _ _ _ w612 _ _ _]
          tunnel: w513 -> [_ _ _ _ _ _ _ _ w623 _ _]
          tunnel: w512 -> [_ _ _ _ _ _ _ _ _ w633 _]
          tunnel: w511 -> [w536 w547 w558 w569 w580 w591 w602 w613 w624 w635 _]
          frame "BIN 1" {
            n119 = Pick Line(multi-line string="TOL\nABS", line index=w540) -> (output string=w539:string)  [unwired: 1 in]
            n120 = property class="Bool"(reference=w535, "Value"=w536) -> ()  [unwired: 1 in, 2 out]
            n121 = Format Into String(format string="%.;:BIN:%s:COMP:BIN1 %d;", w539, w534) -> (resulting string=w542:string)  [unwired: 2 in, 1 out]
            n122 = call "Write.vi"("error in (no error)"=w541, "Input String"=w542, "VISA resource name"=w537) -> ("error out"=w538:errorcluster)  [unwired: 7 in, 1 out]
          }
          frame "BIN 2" {
            n123 = property class="Bool"(reference=w546, "Value"=w547) -> ()  [unwired: 1 in, 2 out]
            n124 = Pick Line(multi-line string="TOL\nABS", line index=w551) -> (output string=w550:string)  [unwired: 1 in]
            n125 = Format Into String(format string="%.;:BIN:%s:COMP:BIN2 %d;", w550, w545) -> (resulting string=w553:string)  [unwired: 2 in, 1 out]
            n126 = call "Write.vi"("error in (no error)"=w552, "Input String"=w553, "VISA resource name"=w548) -> ("error out"=w549:errorcluster)  [unwired: 7 in, 1 out]
          }
          frame "BIN 3" {
            n127 = property class="Bool"(reference=w557, "Value"=w558) -> ()  [unwired: 1 in, 2 out]
            n128 = Pick Line(multi-line string="TOL\nABS", line index=w562) -> (output string=w561:string)  [unwired: 1 in]
            n129 = Format Into String(format string="%.;:BIN:%s:COMP:BIN3 %d;", w561, w556) -> (resulting string=w564:string)  [unwired: 2 in, 1 out]
            n130 = call "Write.vi"("error in (no error)"=w563, "Input String"=w564, "VISA resource name"=w559) -> ("error out"=w560:errorcluster)  [unwired: 7 in, 1 out]
          }
          frame "BIN 4" {
            n131 = property class="Bool"(reference=w568, "Value"=w569) -> ()  [unwired: 1 in, 2 out]
            n132 = Pick Line(multi-line string="TOL\nABS", line index=w573) -> (output string=w572:string)  [unwired: 1 in]
            n133 = Format Into String(format string="%.;:BIN:%s:COMP:BIN4 %d;", w572, w567) -> (resulting string=w575:string)  [unwired: 2 in, 1 out]
            n134 = call "Write.vi"("error in (no error)"=w574, "Input String"=w575, "VISA resource name"=w570) -> ("error out"=w571:errorcluster)  [unwired: 7 in, 1 out]
          }
          frame "BIN 5" {
            n135 = property class="Bool"(reference=w579, "Value"=w580) -> ()  [unwired: 1 in, 2 out]
            n136 = Pick Line(multi-line string="TOL\nABS", line index=w584) -> (output string=w583:string)  [unwired: 1 in]
            n137 = Format Into String(format string="%.;:BIN:%s:COMP:BIN5 %d;", w583, w578) -> (resulting string=w586:string)  [unwired: 2 in, 1 out]
            n138 = call "Write.vi"("error in (no error)"=w585, "Input String"=w586, "VISA resource name"=w581) -> ("error out"=w582:errorcluster)  [unwired: 7 in, 1 out]
          }
          frame "BIN 6" {
            n139 = property class="Bool"(reference=w590, "Value"=w591) -> ()  [unwired: 1 in, 2 out]
            n140 = Pick Line(multi-line string="TOL\nABS", line index=w595) -> (output string=w594:string)  [unwired: 1 in]
            n141 = Format Into String(format string="%.;:BIN:%s:COMP:BIN6 %d;", w594, w589) -> (resulting string=w597:string)  [unwired: 2 in, 1 out]
            n142 = call "Write.vi"("error in (no error)"=w596, "Input String"=w597, "VISA resource name"=w592) -> ("error out"=w593:errorcluster)  [unwired: 7 in, 1 out]
          }
          frame "BIN 7" {
            n143 = property class="Bool"(reference=w601, "Value"=w602) -> ()  [unwired: 1 in, 2 out]
            n144 = Pick Line(multi-line string="TOL\nABS", line index=w606) -> (output string=w605:string)  [unwired: 1 in]
            n145 = Format Into String(format string="%.;:BIN:%s:COMP:BIN7 %d;", w605, w600) -> (resulting string=w608:string)  [unwired: 2 in, 1 out]
            n146 = call "Write.vi"("error in (no error)"=w607, "Input String"=w608, "VISA resource name"=w603) -> ("error out"=w604:errorcluster)  [unwired: 7 in, 1 out]
          }
          frame "BIN 8" {
            n147 = property class="Bool"(reference=w612, "Value"=w613) -> ()  [unwired: 1 in, 2 out]
            n148 = Pick Line(multi-line string="TOL\nABS", line index=w617) -> (output string=w616:string)  [unwired: 1 in]
            n149 = Format Into String(format string="%.;:BIN:%s:COMP:BIN8 %d;", w616, w611) -> (resulting string=w619:string)  [unwired: 2 in, 1 out]
            n150 = call "Write.vi"("error in (no error)"=w618, "Input String"=w619, "VISA resource name"=w614) -> ("error out"=w615:errorcluster)  [unwired: 7 in, 1 out]
          }
          frame "BIN 9" {
            n151 = Pick Line(multi-line string="TOL\nABS", line index=w628) -> (output string=w627:string)  [unwired: 1 in]
            n152 = property class="Bool"(reference=w623, "Value"=w624) -> ()  [unwired: 1 in, 2 out]
            n153 = Format Into String(format string="%.;:BIN:%s:COMP:BIN9 %d;", w627, w622) -> (resulting string=w630:string)  [unwired: 2 in, 1 out]
            n154 = call "Write.vi"("error in (no error)"=w629, "Input String"=w630, "VISA resource name"=w625) -> ("error out"=w626:errorcluster)  [unwired: 7 in, 1 out]
          }
          frame "SEC" {
            n155 = property class="Bool"(reference=w633, "Value"=w635) -> ()  [unwired: 1 in, 2 out]
            n156 = Pick Line(multi-line string="TOL\nABS", line index=w638) -> (output string=w634:string)  [unwired: 1 in]
            n157 = Format Into String(format string="%.;:BIN:%s:COMP:SEC %d;", w634, w641) -> (resulting string=w640:string)  [unwired: 2 in, 1 out]
            n158 = call "Write.vi"("error in (no error)"=w639, "Input String"=w640, "VISA resource name"=w636) -> ("error out"=w637:errorcluster)  [unwired: 7 in, 1 out]
          }
          frame "Default", Default {
          }
        }
      }
      frame "BIN Low Limit" {
        # "Sets the Low limit of the selected BIN."
        n159 = local read "Low Limit Ref"() -> (w649:refnum<vi>)
        n160 = Unbundle By Name(w664) -> ("VISA resource name"=w663:refnum<visa-resource-name>)
        n161 = property on="Property Node" class="DigNum (strict)"(reference=w649) -> ("Label.Text"=w666:string)  [unwired: 1 in, 2 out]
        n162 = local read "Comparator Mode"() -> (w660:u16)
        n163 = local read "New Low Limit Val"() -> (w661:dbl)
        n164 = Unbundle By Name(w648) -> ("BIN 1"=w659:dbl, "BIN 2"=w658:dbl, "BIN 3"=w657:dbl, "BIN 4"=w656:dbl, "BIN 5"=w655:dbl, "BIN 6"=w654:dbl, "BIN 7"=w653:dbl, "BIN 8"=w652:dbl, "BIN 9"=w651:dbl, "SEC"=w650:dbl)
        n165 = case shown="\"BIN 1\"" w666 {
          tunnel: w665 -> [w670 w681 w693 w705 w717 w729 w741 w753 w765 w777 w789]
          tunnel: w663 -> [_ w680 w692 w704 w716 w728 w740 w752 w764 w776 w788]
          tunnel: [w670 w679 w691 w703 w715 w727 w739 w751 w763 w775 w787] -> w662
          tunnel: w661 -> [_ w672 w685 w697 w709 w721 w733 w745 w757 w769 w781]
          tunnel: w660 -> [_ w676 w688 w700 w712 w724 w736 w748 w760 w772 w784]
          tunnel: w659 -> [_ w675 _ _ _ _ _ _ _ _ _]
          tunnel: w658 -> [_ _ w684 _ _ _ _ _ _ _ _]
          tunnel: w657 -> [_ _ _ w696 _ _ _ _ _ _ _]
          tunnel: w656 -> [_ _ _ _ w708 _ _ _ _ _ _]
          tunnel: w655 -> [_ _ _ _ _ w720 _ _ _ _ _]
          tunnel: w654 -> [_ _ _ _ _ _ w732 _ _ _ _]
          tunnel: w653 -> [_ _ _ _ _ _ _ w744 _ _ _]
          tunnel: w652 -> [_ _ _ _ _ _ _ _ w756 _ _]
          tunnel: w651 -> [_ _ _ _ _ _ _ _ _ w768 _]
          tunnel: w650 -> [_ _ _ _ _ _ _ _ _ _ w780]
          tunnel: w647 -> [w671 w674 w687 w699 w711 w723 w735 w747 w759 w771 w783]
          tunnel: [w671 w673 w686 w698 w710 w722 w734 w746 w758 w770 w782] -> w646
          frame "False", Default {
          }
          frame "BIN 1" {
            n166 = Pick Line(multi-line string="TOL\nABS", line index=w676) -> (output string=w678:string)  [unwired: 1 in]
            n167 = Format Into String(format string="%.;:BIN:%s:LIM:BIN1 %g,%g", w678, w672, w675) -> (resulting string=w677:string)  [unwired: 2 in, 1 out]
            n168 = Bundle By Name(cluster=w674, "BIN 1"=w672) -> (w673:T3)
            n169 = call "Write.vi"("error in (no error)"=w681, "Input String"=w677, "VISA resource name"=w680) -> ("error out"=w679:errorcluster)  [unwired: 7 in, 1 out]
          }
          frame "BIN 2" {
            n170 = Pick Line(multi-line string="TOL\nABS", line index=w688) -> (output string=w690:string)  [unwired: 1 in]
            n171 = Format Into String(format string="%.;:BIN:%s:LIM:BIN2 %g,%g", w690, w685, w684) -> (resulting string=w689:string)  [unwired: 2 in, 1 out]
            n172 = Bundle By Name(cluster=w687, "BIN 2"=w685) -> (w686:T3)
            n173 = call "Write.vi"("error in (no error)"=w693, "Input String"=w689, "VISA resource name"=w692) -> ("error out"=w691:errorcluster)  [unwired: 7 in, 1 out]
          }
          frame "BIN 3" {
            n174 = Pick Line(multi-line string="TOL\nABS", line index=w700) -> (output string=w702:string)  [unwired: 1 in]
            n175 = Format Into String(format string="%.;:BIN:%s:LIM:BIN3 %g,%g", w702, w697, w696) -> (resulting string=w701:string)  [unwired: 2 in, 1 out]
            n176 = Bundle By Name(cluster=w699, "BIN 3"=w697) -> (w698:T3)
            n177 = call "Write.vi"("error in (no error)"=w705, "Input String"=w701, "VISA resource name"=w704) -> ("error out"=w703:errorcluster)  [unwired: 7 in, 1 out]
          }
          frame "BIN 4" {
            n178 = Pick Line(multi-line string="TOL\nABS", line index=w712) -> (output string=w714:string)  [unwired: 1 in]
            n179 = Format Into String(format string="%.;:BIN:%s:LIM:BIN4 %g,%g", w714, w709, w708) -> (resulting string=w713:string)  [unwired: 2 in, 1 out]
            n180 = Bundle By Name(cluster=w711, "BIN 4"=w709) -> (w710:T3)
            n181 = call "Write.vi"("error in (no error)"=w717, "Input String"=w713, "VISA resource name"=w716) -> ("error out"=w715:errorcluster)  [unwired: 7 in, 1 out]
          }
          frame "BIN 5" {
            n182 = Pick Line(multi-line string="TOL\nABS", line index=w724) -> (output string=w726:string)  [unwired: 1 in]
            n183 = Format Into String(format string="%.;:BIN:%s:LIM:BIN5 %g,%g", w726, w721, w720) -> (resulting string=w725:string)  [unwired: 2 in, 1 out]
            n184 = Bundle By Name(cluster=w723, "BIN 5"=w721) -> (w722:T3)
            n185 = call "Write.vi"("error in (no error)"=w729, "Input String"=w725, "VISA resource name"=w728) -> ("error out"=w727:errorcluster)  [unwired: 7 in, 1 out]
          }
          frame "BIN 6" {
            n186 = Pick Line(multi-line string="TOL\nABS", line index=w736) -> (output string=w738:string)  [unwired: 1 in]
            n187 = Format Into String(format string="%.;:BIN:%s:LIM:BIN6 %g,%g", w738, w733, w732) -> (resulting string=w737:string)  [unwired: 2 in, 1 out]
            n188 = Bundle By Name(cluster=w735, "BIN 6"=w733) -> (w734:T3)
            n189 = call "Write.vi"("error in (no error)"=w741, "Input String"=w737, "VISA resource name"=w740) -> ("error out"=w739:errorcluster)  [unwired: 7 in, 1 out]
          }
          frame "BIN 7" {
            n190 = Pick Line(multi-line string="TOL\nABS", line index=w748) -> (output string=w750:string)  [unwired: 1 in]
            n191 = Format Into String(format string="%.;:BIN:%s:LIM:BIN7 %g,%g", w750, w745, w744) -> (resulting string=w749:string)  [unwired: 2 in, 1 out]
            n192 = Bundle By Name(cluster=w747, "BIN 7"=w745) -> (w746:T3)
            n193 = call "Write.vi"("error in (no error)"=w753, "Input String"=w749, "VISA resource name"=w752) -> ("error out"=w751:errorcluster)  [unwired: 7 in, 1 out]
          }
          frame "BIN 8" {
            n194 = Pick Line(multi-line string="TOL\nABS", line index=w760) -> (output string=w762:string)  [unwired: 1 in]
            n195 = Format Into String(format string="%.;:BIN:%s:LIM:BIN8 %g,%g", w762, w757, w756) -> (resulting string=w761:string)  [unwired: 2 in, 1 out]
            n196 = Bundle By Name(cluster=w759, "BIN 8"=w757) -> (w758:T3)
            n197 = call "Write.vi"("error in (no error)"=w765, "Input String"=w761, "VISA resource name"=w764) -> ("error out"=w763:errorcluster)  [unwired: 7 in, 1 out]
          }
          frame "BIN 9" {
            n198 = Pick Line(multi-line string="TOL\nABS", line index=w772) -> (output string=w774:string)  [unwired: 1 in]
            n199 = Format Into String(format string="%.;:BIN:%s:LIM:BIN9 %g,%g", w774, w769, w768) -> (resulting string=w773:string)  [unwired: 2 in, 1 out]
            n200 = Bundle By Name(cluster=w771, "BIN 9"=w769) -> (w770:T3)
            n201 = call "Write.vi"("error in (no error)"=w777, "Input String"=w773, "VISA resource name"=w776) -> ("error out"=w775:errorcluster)  [unwired: 7 in, 1 out]
          }
          frame "SEC" {
            n202 = Pick Line(multi-line string="TOL\nABS", line index=w784) -> (output string=w786:string)  [unwired: 1 in]
            n203 = Format Into String(format string="%.;:BIN:%s:LIM:SEC %g,%g", w786, w781, w780) -> (resulting string=w785:string)  [unwired: 2 in, 1 out]
            n204 = call "Write.vi"("error in (no error)"=w789, "Input String"=w785, "VISA resource name"=w788) -> ("error out"=w787:errorcluster)  [unwired: 7 in, 1 out]
            n205 = Bundle By Name(cluster=w783, "SEC"=w781) -> (w782:T3)
          }
        }
      }
      frame "BIN High Limit" {
        # "Sets the High limit of the selected BIN."
        n206 = Unbundle By Name(w811) -> ("VISA resource name"=w810:refnum<visa-resource-name>)
        n207 = local read "New High Limit Val"() -> (w808:dbl)
        n208 = local read "Comparator Mode"() -> (w807:u16)
        n209 = local read "High Limit Ref"() -> (w795:refnum<vi>)
        n210 = property on="Property Node" class="DigNum (strict)"(reference=w795) -> ("Label.Text"=w813:string)  [unwired: 1 in, 2 out]
        n211 = Unbundle By Name(w794) -> ("BIN 1"=w806:dbl, "BIN 2"=w805:dbl, "BIN 3"=w804:dbl, "BIN 4"=w803:dbl, "BIN 5"=w802:dbl, "BIN 6"=w801:dbl, "BIN 7"=w800:dbl, "BIN 8"=w799:dbl, "BIN 9"=w798:dbl, "SEC"=w797:dbl)
        n212 = case shown="\"BIN 2\"" w813 {
          tunnel: w812 -> [w817 w828 w840 w852 w864 w876 w888 w900 w912 w924 w936]
          tunnel: w810 -> [_ w827 w839 w851 w863 w875 w887 w899 w911 w923 w935]
          tunnel: [w817 w826 w838 w850 w862 w874 w886 w898 w910 w922 w934] -> w809
          tunnel: w808 -> [_ w819 w831 w843 w855 w867 w879 w891 w903 w915 w927]
          tunnel: w807 -> [_ w823 w835 w847 w859 w871 w883 w895 w907 w919 w931]
          tunnel: w806 -> [_ w820 _ _ _ _ _ _ _ _ _]
          tunnel: w805 -> [_ _ w832 _ _ _ _ _ _ _ _]
          tunnel: w804 -> [_ _ _ w844 _ _ _ _ _ _ _]
          tunnel: w803 -> [_ _ _ _ w856 _ _ _ _ _ _]
          tunnel: w802 -> [_ _ _ _ _ w868 _ _ _ _ _]
          tunnel: w801 -> [_ _ _ _ _ _ w880 _ _ _ _]
          tunnel: w800 -> [_ _ _ _ _ _ _ w892 _ _ _]
          tunnel: w799 -> [_ _ _ _ _ _ _ _ w904 _ _]
          tunnel: w798 -> [_ _ _ _ _ _ _ _ _ w916 _]
          tunnel: w797 -> [_ _ _ _ _ _ _ _ _ _ w928]
          tunnel: w793 -> [w818 w822 w834 w846 w858 w870 w882 w894 w906 w917 w930]
          tunnel: [w818 w821 w833 w845 w857 w869 w881 w893 w905 w918 w929] -> w792
          frame "False", Default {
          }
          frame "BIN 1" {
            n213 = Pick Line(multi-line string="TOL\nABS", line index=w823) -> (output string=w825:string)  [unwired: 1 in]
            n214 = Format Into String(format string="%.;:BIN:%s:LIM:BIN1 %g,%g", w825, w820, w819) -> (resulting string=w824:string)  [unwired: 2 in, 1 out]
            n215 = Bundle By Name(cluster=w822, "BIN 1"=w819) -> (w821:T3)
            n216 = call "Write.vi"("error in (no error)"=w828, "Input String"=w824, "VISA resource name"=w827) -> ("error out"=w826:errorcluster)  [unwired: 7 in, 1 out]
          }
          frame "BIN 2" {
            n217 = Pick Line(multi-line string="TOL\nABS", line index=w835) -> (output string=w837:string)  [unwired: 1 in]
            n218 = Format Into String(format string="%.;:BIN:%s:LIM:BIN2 %g,%g", w837, w832, w831) -> (resulting string=w836:string)  [unwired: 2 in, 1 out]
            n219 = Bundle By Name(cluster=w834, "BIN 2"=w831) -> (w833:T3)
            n220 = call "Write.vi"("error in (no error)"=w840, "Input String"=w836, "VISA resource name"=w839) -> ("error out"=w838:errorcluster)  [unwired: 7 in, 1 out]
          }
          frame "BIN 3" {
            n221 = Pick Line(multi-line string="TOL\nABS", line index=w847) -> (output string=w849:string)  [unwired: 1 in]
            n222 = Format Into String(format string="%.;:BIN:%s:LIM:BIN3 %g,%g", w849, w844, w843) -> (resulting string=w848:string)  [unwired: 2 in, 1 out]
            n223 = Bundle By Name(cluster=w846, "BIN 3"=w843) -> (w845:T3)
            n224 = call "Write.vi"("error in (no error)"=w852, "Input String"=w848, "VISA resource name"=w851) -> ("error out"=w850:errorcluster)  [unwired: 7 in, 1 out]
          }
          frame "BIN 4" {
            n225 = Pick Line(multi-line string="TOL\nABS", line index=w859) -> (output string=w861:string)  [unwired: 1 in]
            n226 = Format Into String(format string="%.;:BIN:%s:LIM:BIN4 %g,%g", w861, w856, w855) -> (resulting string=w860:string)  [unwired: 2 in, 1 out]
            n227 = Bundle By Name(cluster=w858, "BIN 4"=w855) -> (w857:T3)
            n228 = call "Write.vi"("error in (no error)"=w864, "Input String"=w860, "VISA resource name"=w863) -> ("error out"=w862:errorcluster)  [unwired: 7 in, 1 out]
          }
          frame "BIN 5" {
            n229 = Pick Line(multi-line string="TOL\nABS", line index=w871) -> (output string=w873:string)  [unwired: 1 in]
            n230 = Format Into String(format string="%.;:BIN:%s:LIM:BIN5 %g,%g", w873, w868, w867) -> (resulting string=w872:string)  [unwired: 2 in, 1 out]
            n231 = Bundle By Name(cluster=w870, "BIN 5"=w867) -> (w869:T3)
            n232 = call "Write.vi"("error in (no error)"=w876, "Input String"=w872, "VISA resource name"=w875) -> ("error out"=w874:errorcluster)  [unwired: 7 in, 1 out]
          }
          frame "BIN 6" {
            n233 = Pick Line(multi-line string="TOL\nABS", line index=w883) -> (output string=w885:string)  [unwired: 1 in]
            n234 = Format Into String(format string="%.;:BIN:%s:LIM:BIN6 %g,%g", w885, w880, w879) -> (resulting string=w884:string)  [unwired: 2 in, 1 out]
            n235 = Bundle By Name(cluster=w882, "BIN 6"=w879) -> (w881:T3)
            n236 = call "Write.vi"("error in (no error)"=w888, "Input String"=w884, "VISA resource name"=w887) -> ("error out"=w886:errorcluster)  [unwired: 7 in, 1 out]
          }
          frame "BIN 7" {
            n237 = Pick Line(multi-line string="TOL\nABS", line index=w895) -> (output string=w897:string)  [unwired: 1 in]
            n238 = Format Into String(format string="%.;:BIN:%s:LIM:BIN7 %g,%g", w897, w892, w891) -> (resulting string=w896:string)  [unwired: 2 in, 1 out]
            n239 = Bundle By Name(cluster=w894, "BIN 7"=w891) -> (w893:T3)
            n240 = call "Write.vi"("error in (no error)"=w900, "Input String"=w896, "VISA resource name"=w899) -> ("error out"=w898:errorcluster)  [unwired: 7 in, 1 out]
          }
          frame "BIN 8" {
            n241 = Pick Line(multi-line string="TOL\nABS", line index=w907) -> (output string=w909:string)  [unwired: 1 in]
            n242 = Format Into String(format string="%.;:BIN:%s:LIM:BIN8 %g,%g", w909, w904, w903) -> (resulting string=w908:string)  [unwired: 2 in, 1 out]
            n243 = Bundle By Name(cluster=w906, "BIN 8"=w903) -> (w905:T3)
            n244 = call "Write.vi"("error in (no error)"=w912, "Input String"=w908, "VISA resource name"=w911) -> ("error out"=w910:errorcluster)  [unwired: 7 in, 1 out]
          }
          frame "BIN 9" {
            n245 = Pick Line(multi-line string="TOL\nABS", line index=w919) -> (output string=w921:string)  [unwired: 1 in]
            n246 = Format Into String(format string="%.;:BIN:%s:LIM:BIN9 %g,%g", w921, w916, w915) -> (resulting string=w920:string)  [unwired: 2 in, 1 out]
            n247 = Bundle By Name(cluster=w917, "BIN 9"=w915) -> (w918:T3)
            n248 = call "Write.vi"("error in (no error)"=w924, "Input String"=w920, "VISA resource name"=w923) -> ("error out"=w922:errorcluster)  [unwired: 7 in, 1 out]
          }
          frame "SEC" {
            n249 = Pick Line(multi-line string="TOL\nABS", line index=w931) -> (output string=w933:string)  [unwired: 1 in]
            n250 = Format Into String(format string="%.;:BIN:%s:LIM:SEC %g,%g", w933, w928, w927) -> (resulting string=w932:string)  [unwired: 2 in, 1 out]
            n251 = call "Write.vi"("error in (no error)"=w936, "Input String"=w932, "VISA resource name"=w935) -> ("error out"=w934:errorcluster)  [unwired: 7 in, 1 out]
            n252 = Bundle By Name(cluster=w930, "SEC"=w927) -> (w929:T3)
          }
        }
      }
      frame "BIN Nominal" {
        # "Sets nomial value for tolerance mode."
        n253 = local read "Comparator Mode"() -> (w942:u16)
        n254 = Unbundle By Name(w940) -> ("VISA resource name"=w939:refnum<visa-resource-name>)
        n255 = Equal To 0?(x=w942) -> (x = 0?=w941:bool)
        n256 = case shown="False" w941 {
          tunnel: w945 -> [w953 w960]
          tunnel: [w953 w959] -> w944
          tunnel: w939 -> [_ w955]
          frame False {
            n257 = local read "OldVal"() -> (w951:dbl)
            n258 = local read "CtlRef"() -> (w952:refnum<vi>)
            n259 = property class="DigNum (strict)"(reference=w952, "Value"=w951) -> ()  [unwired: 1 in, 2 out]
            n260 = One Button Dialog(message="Nominal Value is only available for\nTolerance Mode. Please select tolerance \nand then input the Nominal value.\n") -> ()  [unwired: 1 in, 1 out]
          }
          frame True {
            n261 = Format Into String(format string="%.;:BIN:TOL:NOM %g;", "Nominal Value (0.0)") -> (resulting string=w956:string)  [unwired: 2 in, 1 out]
            n262 = call "Write.vi"("error in (no error)"=w960, "Input String"=w956, "VISA resource name"=w955) -> ("error out"=w959:errorcluster)  [unwired: 7 in, 1 out]
          }
        }
      }
      frame "BIN Config" {
        w976 = UI_State."Idle"  # UI State
        # "Configure the Function and Mode of the selected BIN."
        n263 = Unbundle By Name(w965) -> ("VISA resource name"=w972:refnum<visa-resource-name>)
        n264 = local read "Comparator Mode"() -> (w963:u16)
        n265 = local read "Function"() -> (w971:u16)
        n266 = call "Configure Comparator Mode.vi"("Comparator Mode (1:Absolute)"=w963, "error in (no error)"=w970, "Function (4: Cp-D)"=w971, "Display Mode (0:BIN)"="Bin Display Mode", "VISA resource name"=w972) -> ("error out"=w967:errorcluster)  [unwired: 5 in, 1 out]
        n267 = Bundle By Name(cluster=w965, "Comparator Mode"=w963) -> (w964:T8)
        n268 = call-poly "Enqueue Message.vi"("error in (no error)"=w967, "Message"="Update Settings", "Message Queue"=w968) -> ("error out"=w966:errorcluster)  [unwired: 7 in, 1 out]
      }
      frame "Beeper Mode" {
        # "Set the beeper mode for when the comparator fails or passes."
        n269 = Unbundle By Name(w980) -> ("VISA resource name"=w983:refnum<visa-resource-name>)
        n270 = call "Configure Comparator Beeper.vi"("error in (no error)"=w985, "Beeper Mode (2: Beep when Failed)"="Beeper Mode", "VISA resource name"=w983) -> ("error out"=w984:errorcluster)  [unwired: 7 in, 1 out]
      }
      frame "BIN Count" {
        # "\"Enable BIN Count\""
        n271 = Unbundle By Name(w998) -> ("VISA resource name"=w996:refnum<visa-resource-name>)
        n272 = call "Enable Bin Counting.vi"("Enable Bin Count State (T:Enable)"="Count State", "error in (no error)"=w995, "VISA resource name"=w996) -> ("error out"=w991:errorcluster)  [unwired: 7 in, 1 out]
        n273 = case shown="False" "Count State" {
          tunnel: w991 -> [w1003 w1008]
          tunnel: [w1003 w1007] -> w990
          tunnel: w989 -> [_ w1006]
          frame False {
            w1004 = T10."Enabled" ("Disabled")
            n274 = property on="Comparator Swap" class="Bool (strict)"("DisabledEnum"=w1004) -> ()  [unwired: 2 in, 2 out]
            n275 = property on="Clear Count" class="Bool (strict)"("DisabledEnum"=w1004) -> ()  [unwired: 2 in, 2 out]
            n276 = property on="Trigger" class="Bool (strict)"("DisabledEnum"=T10."Disabled and Grayed Out" ("Disabled")) -> ()  [unwired: 2 in, 2 out]
          }
          frame True {
            w1010 = T10."Disabled and Grayed Out" ("Disabled")
            n277 = call-poly "Enqueue Message.vi"("error in (no error)"=w1008, "Message"="BIN Read", "Message Queue"=w1006) -> ("error out"=w1007:errorcluster)  [unwired: 7 in, 1 out]
            n278 = property on="Comparator Swap" class="Bool (strict)"("DisabledEnum"=w1010) -> ()  [unwired: 2 in, 2 out]
            n279 = property on="Clear Count" class="Bool (strict)"("DisabledEnum"=w1010) -> ()  [unwired: 2 in, 2 out]
            n280 = property on="Trigger" class="Bool (strict)"("DisabledEnum"=T10."Enabled" ("Disabled")) -> ()  [unwired: 2 in, 2 out]
          }
        }
        n281 = Wait (ms)(milliseconds to wait=u32 100) -> ()  [unwired: 1 out]
      }
      frame "Comparator  Swap" {
        # "\"Swap betweeen the primary and secondary measurement?\""
        n282 = Unbundle By Name(w1014) -> ("VISA resource name"=w1018:refnum<visa-resource-name>)
        n283 = call "Configure Comparator Swap.vi"("error in (no error)"=w1019, "Enable Comparator Swap (F:Disable)"="Comparator Swap", "VISA resource name"=w1018) -> ("error out"=w1016:errorcluster)  [unwired: 7 in, 1 out]
      }
      frame "Trigger BIN" {
        # "Sends a BUS trigger to trigger a single BIN count."
        n284 = Unbundle By Name(w1031) -> ("VISA resource name"=w1030:refnum<visa-resource-name>)
        n285 = call "Send Software Trigger.vi"("error in (no error)"=w1029, "VISA resource name"=w1030) -> ("error out"=w1026:errorcluster)  [unwired: 8 in, 1 out]
        n286 = call-poly "Enqueue Message.vi"("error in (no error)"=w1026, "Message"="BIN Read", "Message Queue"=w1027) -> ("error out"=w1025:errorcluster)  [unwired: 7 in, 1 out]
      }
      frame "BIN Clear" {
        # "Clears the BIN count."
        n287 = Unbundle By Name(w1042) -> ("VISA resource name"=w1046:refnum<visa-resource-name>)
        n288 = local read "Comparator Mode"() -> (w1044:u16)
        n289 = call "Clear Comparator Bin Count.vi"("error in (no error)"=w1047, "Comparator Mode (1:Absolute)"=w1044, "VISA resource name"=w1046) -> ("error out"=w1038:errorcluster)  [unwired: 7 in, 1 out]
        n290 = call-poly "Enqueue Message.vi"("error in (no error)"=w1038, "Message"="BIN Read", "Message Queue"=w1036) -> ("error out"=w1037:errorcluster)  [unwired: 7 in, 1 out]
      }
      frame "Enable Sweep" {
        # "Enables the sweep and disables the parameters: Function, Range, Speed, Level, and Frequency."
        n291 = local read "Enable Sweep New Value"() -> (w1050:bool)
        n292 = Unbundle By Name(w1059) -> ("VISA resource name"=w1057:refnum<visa-resource-name>)
        n293 = case shown="True" w1050 {
          tunnel: [w1084 w1110] -> w1061
          tunnel: w1058 -> [w1083 w1119]
          tunnel: w1057 -> [w1082 w1111]
          tunnel: w1056 -> [w1068 w1122]
          tunnel: w1052 -> [w1066 w1112]
          tunnel: w1051 -> [w1064 w1113]
          frame True {
            n294 = flat-sequence {
              tunnel: w1083 -> [w1093]
              tunnel: [w1092] -> w1087
              tunnel: w1066 -> [w1089]
              tunnel: [w1088] -> w1065
              tunnel: w1064 -> [w1088]
              tunnel: [w1101] -> w1086
              tunnel: w1087 -> [w1099]
              tunnel: w1082 -> [w1094]
              tunnel: [w1100] -> w1085
              tunnel: w1065 -> [w1095]
              tunnel: [w1095] -> w1063
              tunnel: [w1106] -> w1084
              tunnel: w1086 -> [w1109]
              tunnel: w1085 -> [w1108]
              tunnel: w1063 -> [w1102]
              frame #0 {
                n295 = Wait (ms)(milliseconds to wait=u32 1000) -> ()  [unwired: 1 out]
                n296 = call-poly "Enqueue Message.vi"("error in (no error)"=w1093, "Message"="Stop", "Message Queue"=w1089) -> ("error out"=w1092:errorcluster)  [unwired: 7 in, 1 out]
              }
              frame #1 {
                n297 = call-poly "Enqueue Message.vi"("error in (no error)"=w1099, "Message Data"="Running Sweep" ("Message"), "Message"="Update Status", "Message Queue"=w1095) -> ("error out"=w1098:errorcluster)  [unwired: 6 in, 1 out]
                n298 = VISA Open(error in (no error)=w1098, VISA resource name=w1094) -> (VISA resource name=w1100:refnum<visa-resource-name>, error out=w1101:errorcluster)  [unwired: 3 in]
              }
              frame #2 {
                n299 = call "Write.vi"("error in (no error)"=w1109, "Input String"="SWEE:STAR 1" ("format string"), "VISA resource name"=w1108) -> ("error out"=w1107:errorcluster)  [unwired: 7 in, 1 out]
                n300 = call-poly "Enqueue Message.vi"("error in (no error)"=w1107, "Message"="Running Sweep", "Message Queue"=w1102) -> ("error out"=w1106:errorcluster)  [unwired: 7 in, 1 out]
                n301 = Wait (ms)(milliseconds to wait=u32 13000) -> ()  [unwired: 1 out]
              }
            }
            n302 = Unbundle By Name(w1068) -> ("Sweep Mode Ref"=w1076:refnum<vi>, "Sweep Display Mode Ref"=w1077:refnum<vi>, "Sweep Parameter Ref"=w1078:refnum<vi>, "Interporlation Ref"=w1079:refnum<vi>, "Sweep Step Ref"=w1080:refnum<vi>, "Autoscale Sweep"=w1081:refnum<vi>, "Start Freq Ref"=w1075:refnum<vi>, "Stop Freq Ref"=w1074:refnum<vi>, "Autoscale Frequency"=w1073:refnum<vi>, "Sweep Low Limit Ref"=w1072:refnum<vi>, "Sweep High Limit Ref"=w1071:refnum<vi>)
            n303 = Build Array(w1076, w1077, w1078, w1079, w1080, w1081, w1075, w1074, w1073, w1072, w1071) -> (w1070:refnum<vi>[])
            n304 = call "Set Enable State on Multiple Controls.vi"("Enable?"=FALSE, "Controls"=w1070) -> ()  [unwired: 10 in]
            n305 = One Button Dialog(message="Please Wait for the Sweep to complete. \n") -> ()  [unwired: 1 in, 1 out]
          }
          frame False {
            n306 = Unbundle By Name(w1122) -> ("Sweep Mode Ref"=w1130:refnum<vi>, "Sweep Display Mode Ref"=w1131:refnum<vi>, "Sweep Parameter Ref"=w1132:refnum<vi>, "Interporlation Ref"=w1133:refnum<vi>, "Sweep Step Ref"=w1134:refnum<vi>, "Autoscale Sweep"=w1135:refnum<vi>, "Start Freq Ref"=w1129:refnum<vi>, "Stop Freq Ref"=w1128:refnum<vi>, "Autoscale Frequency"=w1127:refnum<vi>, "Sweep Low Limit Ref"=w1126:refnum<vi>, "Sweep High Limit Ref"=w1125:refnum<vi>)
            n307 = Build Array(w1130, w1131, w1132, w1133, w1134, w1135, w1129, w1128, w1127, w1126, w1125) -> (w1124:refnum<vi>[])
            n308 = call "Write.vi"("error in (no error)"=w1119, "Input String"="SWEE:STAR 0" ("format string"), "VISA resource name"=w1111) -> ("error out"=w1114:errorcluster)  [unwired: 7 in, 1 out]
            n309 = call "Set Enable State on Multiple Controls.vi"("Enable?"=TRUE, "Controls"=w1124) -> ()  [unwired: 10 in]
            n310 = call-poly "Enqueue Message.vi"("error in (no error)"=w1114, "Message Data"="Acquiring" ("Message"), "Message"="Update Status", "Message Queue"=w1113) -> ("error out"=w1117:errorcluster)  [unwired: 6 in, 1 out]
            n311 = One Button Dialog(message="Sweep has been stopped.") -> ()  [unwired: 1 in, 1 out]
            n312 = call-poly "Enqueue Message.vi"("error in (no error)"=w1117, "Message"="Start", "Message Queue"=w1112) -> ("error out"=w1110:errorcluster)  [unwired: 7 in, 1 out]
          }
        }
      }
      frame "Sweep Function" {
        # "Select function"
        # "Sets the sweep's function"
        n313 = local read "Sweep Display Mode"() -> (w1138:u16)
        n314 = local read "Sweep Mode"() -> (w1149:u16)
        n315 = Unbundle By Name(w1143) -> ("VISA resource name"=w1142:refnum<visa-resource-name>)
        n316 = Pick Line(multi-line string="GRAP\nTAB", line index=w1138) -> (output string=w1140:string)  [unwired: 1 in]
        n317 = Pick Line(multi-line string="LIN\nLOG", line index=w1149) -> (output string=w1148:string)  [unwired: 1 in]
        n318 = Format Into String(w1140) -> (resulting string=w1139:string)  [unwired: 3 in, 1 out]
        n319 = Format Into String(format string="%.;:SWEEP:DISP:%s:%s %d", w1148, w1139, "Sweep Function") -> (resulting string=w1152:string)  [unwired: 2 in, 1 out]
        n320 = call "Write.vi"("error in (no error)"=w1147, "Input String"=w1152, "VISA resource name"=w1142) -> ("error out"=w1146:errorcluster)  [unwired: 7 in, 1 out]
      }
      frame "Sweep Mode" {
        # "Sets the Sweep display mode."
        n321 = Unbundle By Name(w1159) -> ("VISA resource name"=w1158:refnum<visa-resource-name>)
        n322 = Pick Line(multi-line string="LIN\nLOG", line index="Sweep Mode") -> (output string=w1164:string)  [unwired: 1 in]
        n323 = Format Into String(format string="SWEE:MODE %s" ("string (\"\")"), w1164) -> (resulting string=w1165:string)  [unwired: 2 in, 1 out]
        n324 = call "Write.vi"("error in (no error)"=w1163, "Input String"=w1165, "VISA resource name"=w1158) -> ("error out"=w1162:errorcluster)  [unwired: 7 in, 1 out]
      }
      frame "Sweep Swap" {
        # "Select parameter"
        # "Selects either primary or secondary parameter for the sweep."
        n325 = Unbundle By Name(w1176) -> ("VISA resource name"=w1174:refnum<visa-resource-name>)
        n326 = Format Into String(format string="%.;SWEE:SWAP %d\n", "Sweep Parameter") -> (resulting string=w1178:string)  [unwired: 2 in, 1 out]
        n327 = call "Write.vi"("error in (no error)"=w1175, "Input String"=w1178, "VISA resource name"=w1174) -> ("error out"=w1173:errorcluster)  [unwired: 7 in, 1 out]
      }
      frame "Sweep Interpolation" {
        # "Enable interpolation"
        # "Sets the interpolation. Disables and grays out Sweep Step if enabled."
        n328 = local read "Interpolation"() -> (w1185:u16)
        n329 = Unbundle By Name(w1187) -> ("Sweep Step Ref"=w1186:refnum<vi>)
        n330 = Unbundle By Name(w1193) -> ("VISA resource name"=w1192:refnum<visa-resource-name>)
        n331 = Format Into String(format string="SWEE:INTERP %d", w1185) -> (resulting string=w1190:string)  [unwired: 2 in, 1 out]
        n332 = Equal To 0?(x=w1185) -> (x = 0?=w1184:bool)
        n333 = case shown="True" w1184 {
          tunnel: w1186 -> [w1199 w1202]
          frame False {
            n334 = property class="Ring"(reference=w1199, "DisabledEnum"=T10."Disabled and Grayed Out" ("Disabled")) -> ()  [unwired: 1 in, 2 out]
          }
          frame True {
            n335 = property class="Ring"(reference=w1202, "DisabledEnum"=T10."Enabled" ("Disabled")) -> ()  [unwired: 1 in, 2 out]
          }
        }
        n336 = call "Write.vi"("error in (no error)"=w1195, "Input String"=w1190, "VISA resource name"=w1192) -> ("error out"=w1194:errorcluster)  [unwired: 7 in, 1 out]
      }
      frame "Sweep Step" {
        # "Sets sweep step"
        # "Sets the step of the sweep"
        n337 = local read "Sweep Points"() -> (w1208:i32)
        n338 = Unbundle By Name(w1207) -> ("VISA resource name"=w1206:refnum<visa-resource-name>)
        n339 = Pick Line(multi-line string="1\n2\n5\n10", line index=w1208) -> (output string=w1214:string)  [unwired: 1 in]
        n340 = Format Into String(format string="%.;:SWEE:STEP %s\n", w1214) -> (resulting string=w1211:string)  [unwired: 2 in, 1 out]
        n341 = call "Write.vi"("error in (no error)"=w1210, "Input String"=w1211, "VISA resource name"=w1206) -> ("error out"=w1209:errorcluster)  [unwired: 7 in, 1 out]
      }
      frame "Sweep Frequency Autoscale" {
        # "Enable/disable autoscale frequency"
        # "Enable/disables frequency autoscale of sweep."
        n342 = Unbundle By Name(w1222) -> ("VISA resource name"=w1221:refnum<visa-resource-name>)
        n343 = Format Into String(format string=":SWEE:AUTO:FREQ %d\n", "Autoscale Frequency") -> (resulting string=w1225:string)  [unwired: 2 in, 1 out]
        n344 = call "Write.vi"("error in (no error)"=w1224, "Input String"=w1225, "VISA resource name"=w1221) -> ("error out"=w1223:errorcluster)  [unwired: 7 in, 1 out]
        n345 = case shown="False" "Autoscale Frequency" {
          frame False {
            w1231 = T10."Enabled" ("Disabled")
            n346 = property on="Start Frequency" class="DigNum (strict)"("DisabledEnum"=w1231) -> ()  [unwired: 2 in, 2 out]
            n347 = property on="Stop Frequency" class="DigNum (strict)"("DisabledEnum"=w1231) -> ()  [unwired: 2 in, 2 out]
          }
          frame True {
            w1232 = T10."Disabled and Grayed Out" ("Disabled")
            n348 = property on="Start Frequency" class="DigNum (strict)"("DisabledEnum"=w1232) -> ()  [unwired: 2 in, 2 out]
            n349 = property on="Stop Frequency" class="DigNum (strict)"("DisabledEnum"=w1232) -> ()  [unwired: 2 in, 2 out]
          }
        }
      }
      frame "Sweep Range" {
        # "Sets the start and stop frequency of the sweep if frequency autoscale is disabled."
        n350 = Unbundle By Name(w1236) -> ("VISA resource name"=w1235:refnum<visa-resource-name>)
        n351 = Format Into String(format string="%.;:SWEE:FREQ:STAR %.1f;:SWEE:FREQ:STOP %.1f\n\n", "Start Frequency", "Stop Frequency") -> (resulting string=w1240:string)  [unwired: 2 in, 1 out]
        n352 = call "Write.vi"("Input String"=w1240, "VISA resource name"=w1235) -> ()  [unwired: 8 in, 2 out]
      }
      frame "Sweep Limit Autoscale" {
        # "Enable/disable autoscale"
        # "Enable/disable the sweep's limit autoscale"
        n353 = Unbundle By Name(w1250) -> ("VISA resource name"=w1249:refnum<visa-resource-name>)
        n354 = Format Into String(format string=":SWEE:AUTO:SCAL %d\n", "Autoscale Limit") -> (resulting string=w1253:string)  [unwired: 2 in, 1 out]
        n355 = call "Write.vi"("error in (no error)"=w1252, "Input String"=w1253, "VISA resource name"=w1249) -> ("error out"=w1251:errorcluster)  [unwired: 7 in, 1 out]
        n356 = case shown="True" "Autoscale Limit" {
          frame False {
            w1259 = T10."Enabled" ("Disabled")
            n357 = property on="Sweep High Limit" class="DigNum (strict)"("DisabledEnum"=w1259) -> ()  [unwired: 2 in, 2 out]
            n358 = property on="Sweep Low Limit" class="DigNum (strict)"("DisabledEnum"=w1259) -> ()  [unwired: 2 in, 2 out]
          }
          frame True {
            w1260 = T10."Disabled and Grayed Out" ("Disabled")
            n359 = property on="Sweep High Limit" class="DigNum (strict)"("DisabledEnum"=w1260) -> ()  [unwired: 2 in, 2 out]
            n360 = property on="Sweep Low Limit" class="DigNum (strict)"("DisabledEnum"=w1260) -> ()  [unwired: 2 in, 2 out]
          }
        }
      }
      frame "Sweep Limit Range" {
        w1265 = "%.;:SWEE:DISP:LIM %f,%f\n"  # Sets the limit values
        # "Sets the value limit on the sweep display."
        n361 = Unbundle By Name(w1270) -> ("VISA resource name"=w1266:refnum<visa-resource-name>)
        n362 = Format Into String(format string=w1265, "Sweep Low Limit", "Sweep High Limit") -> (resulting string=w1269:string)  [unwired: 2 in, 1 out]
        n363 = call "Write.vi"("error in (no error)"=w1268, "Input String"=w1269, "VISA resource name"=w1266) -> ("error out"=w1267:errorcluster)  [unwired: 7 in, 1 out]
      }
      frame "Sweep Display Mode" {
        # "Set sweep display"
        n364 = local read "Sweep Display Mode"() -> (w1283:u16)
        n365 = Unbundle By Name(w1278) -> ("VISA resource name"=w1277:refnum<visa-resource-name>)
        n366 = Pick Line(multi-line string="GRAP\nTAB", line index=w1283) -> (output string=w1285:string)  [unwired: 1 in]
        n367 = Format Into String(format string="%.;:SWEE:DISP:MODE %s", w1285) -> (resulting string=w1284:string)  [unwired: 2 in, 1 out]
        n368 = call "Write.vi"("error in (no error)"=w1282, "Input String"=w1284, "VISA resource name"=w1277) -> ("error out"=w1281:errorcluster)  [unwired: 7 in, 1 out]
      }
      frame "Running Sweep" {
        w1300 = UI_State."Waiting for Sweep(Sweep Complete)"  # UI State
        # "Checks if the sweep is still running."
        n369 = flat-sequence {
          tunnel: w1298 -> [w1304]
          tunnel: w1297 -> [w1303]
          tunnel: [w1302] -> w1295
          tunnel: w1296 -> [w1328]
          tunnel: w1295 -> [w1327]
          tunnel: [w1326] -> w1294
          frame #0 {
            n370 = while {
              tunnel: w1303 -> [w1307]
              tunnel: [w1309] -> w1302
              tunnel: w1304 -> [w1308]
              stop <- w1306 stop-if-true
              n371 = local read "Enable Sweep New Value"() -> (w1305:bool)
              n372 = case shown="False" w1305 {
                selector: w1305 -> [w1312 _]
                tunnel: [w1310 w1321] -> w1309
                tunnel: w1308 -> [w1310 w1315]
                tunnel: w1307 -> [_ w1314]
                tunnel: [w1311 w1313] -> w1306
                frame False {
                  n373 = Not(x=w1312) -> (.not. x?=w1311:bool)
                }
                frame True {
                  n374 = call "Write.vi"("error in (no error)"=w1315, "Input String"="SWEE:BUSY?", "VISA resource name"=w1314) -> ("error out"=w1324:errorcluster, "VISA resource name out"=w1323:refnum<visa-resource-name>)  [unwired: 7 in]
                  n375 = VISA Read(VISA resource name=w1323, byte count=u32 256, error in (no error)=w1324) -> (read buffer=w1319:string, error out=w1321:errorcluster)  [unwired: 2 out]
                  n376 = Match Pattern(string=w1319, regular expression="OFF" ("y")) -> (offset past match=w1318:i32)  [unwired: 1 in, 3 out]
                  n377 = Greater Or Equal To 0?(x=w1318) -> (x >= 0?=w1313:bool)
                  n378 = Wait (ms)(milliseconds to wait=u32 500) -> ()  [unwired: 1 out]
                }
              }
            }
          }
          frame #1 {
            n379 = call-poly "Enqueue Message.vi"("error in (no error)"=w1327, "Message"="Plot Sweep", "Message Queue"=w1328) -> ("error out"=w1326:errorcluster)  [unwired: 7 in, 1 out]
          }
        }
        n380 = Unbundle By Name(w1292) -> ("VISA resource name"=w1297:refnum<visa-resource-name>)
      }
      frame "Plot Sweep" {
        # "Plots the sweep once the sweep is complete, and reables data acquisition."
        n381 = local read "Interpolation"() -> (w1358:u16)
        n382 = Unbundle By Name(w1355) -> ("Enable Sweep"=w1341:refnum<vi>, "Sweep Mode Ref"=w1349:refnum<vi>, "Sweep Display Mode Ref"=w1350:refnum<vi>, "Sweep Parameter Ref"=w1351:refnum<vi>, "Interporlation Ref"=w1352:refnum<vi>, "Sweep Step Ref"=w1353:refnum<vi>, "Autoscale Sweep"=w1354:refnum<vi>, "Start Freq Ref"=w1348:refnum<vi>, "Stop Freq Ref"=w1347:refnum<vi>, "Autoscale Frequency"=w1346:refnum<vi>, "Sweep Low Limit Ref"=w1345:refnum<vi>, "Sweep High Limit Ref"=w1344:refnum<vi>)
        n383 = local read "Sweep Points"() -> (w1359:i32)
        n384 = Unbundle By Name(w1356) -> ("VISA resource name"=w1362:refnum<visa-resource-name>)
        n385 = flat-sequence {
          tunnel: w1363 -> [w1369]
          tunnel: w1358 -> [w1367]
          tunnel: w1359 -> [w1366]
          tunnel: w1362 -> [w1365]
          tunnel: [w1368] -> w1361
          tunnel: [w1372] -> w1334
          tunnel: w1361 -> [w1374]
          tunnel: w1333 -> [w1373]
          frame #0 {
            n386 = call "Sweep Point Acquire.vi"("error in (no error)"=w1369, "Sweep Step"=w1366, "Interpolation"=w1367, "VISA Resource Name"=w1365) -> ("error out"=w1368:errorcluster, "Cluster"=→"XY Graph":cluster{"Array":dbl[], "Array":dbl[]})  [unwired: 5 in, 1 out]
            n387 = Wait (ms)(milliseconds to wait=u32 1000) -> ()  [unwired: 1 out]
          }
          frame #1 {
            n388 = call-poly "Enqueue Message.vi"("error in (no error)"=w1374, "Message"="Broadcast Settings", "Message Queue"=w1373) -> ("error out"=w1372:errorcluster)  [unwired: 7 in, 1 out]
            n389 = One Button Dialog(message="Sweep Complete") -> ()  [unwired: 1 in, 1 out]
          }
        }
        n390 = Build Array(w1349, w1350, w1351, w1352, w1353, w1354, w1348, w1347, w1346, w1345, w1344) -> (w1343:refnum<vi>[])
        n391 = property class="Bool"(reference=w1341, "Value"=FALSE ("Enable?")) -> ()  [unwired: 1 in, 2 out]
        n392 = call "Set Enable State on Multiple Controls.vi"("Enable?"=TRUE, "Controls"=w1343) -> ()  [unwired: 10 in]
        n393 = call-poly "Enqueue Message.vi"("error in (no error)"=w1334, "Message Data"="Acquiring" ("Message"), "Message"="Update Status", "Message Queue"=w1333) -> ("error out"=w1335:errorcluster)  [unwired: 6 in, 1 out]
        n394 = call-poly "Enqueue Message.vi"("error in (no error)"=w1335, "Message"="Start", "Message Queue"=w1337) -> ("error out"=w1336:errorcluster)  [unwired: 7 in, 1 out]
      }
      frame "Start" {
        # "Starts data logging."
        n395 = Unbundle By Name(w1396) -> ("Stop Ref"=w1391:refnum<vi>, "Start Ref"=w1390:refnum<vi>, "Exit Ref"=w1389:refnum<vi>, "Settings Ref"=w1388:refnum<vi>)
        n396 = Build Array(w1391) -> (w1393:refnum<vi>[])
        n397 = Build Array(w1390, w1389, w1388) -> (w1394:refnum<vi>[])
        n398 = call-poly "Enqueue Message.vi"("error in (no error)"=w1398, "Message Data"="Acquiring and Logging..." ("Acquiring and Logging..."), "Message"="Update Status", "Message Queue"=w1380) -> ("error out"=w1387:errorcluster)  [unwired: 6 in, 1 out]
        n399 = call "Set Enable State on Multiple Controls.vi"("Enable?"=FALSE, "Controls"=w1394) -> ()  [unwired: 10 in]
        n400 = call "Set Enable State on Multiple Controls.vi"("Enable?"=TRUE, "Controls"=w1393) -> ()  [unwired: 10 in]
        n401 = call-poly "Enqueue Message.vi"("error in (no error)"=w1387, "Message"="Start", "Message Queue"=w1386) -> ("error out"=w1382:errorcluster)  [unwired: 7 in, 1 out]
      }
      frame "Stop" {
        # "Stops data logging."
        n402 = call-poly "Enqueue Message.vi"("error in (no error)"=w1418, "Message"="Stop", "Message Queue"=w1407) -> ("error out"=w1403:errorcluster)  [unwired: 7 in, 1 out]
        n403 = Unbundle By Name(w1417) -> ("Stop Ref"=w1412:refnum<vi>, "Start Ref"=w1411:refnum<vi>, "Exit Ref"=w1410:refnum<vi>, "Settings Ref"=w1409:refnum<vi>)
        n404 = Build Array(w1412) -> (w1414:refnum<vi>[])
        n405 = Build Array(w1411, w1410, w1409) -> (w1415:refnum<vi>[])
        n406 = call "Set Enable State on Multiple Controls.vi"("Enable?"=TRUE, "Controls"=w1415) -> ()  [unwired: 10 in]
        n407 = call "Set Enable State on Multiple Controls.vi"("Enable?"=FALSE, "Controls"=w1414) -> ()  [unwired: 10 in]
        n408 = case shown="Default" w1405 {
          selector: w1405 -> [w1419 _]
          tunnel: [w1419 UI_State."Waiting for Stop" ("UI State")] -> w1406
          frame "Waiting for Exit" {
          }
          frame Default {
          }
        }
      }
      frame "Acquisition Stopped" {
        # "Logic for determining what action to take when the acquisition has stopped."
        n409 = case shown="Default" w1430 {
          selector: w1430 -> [w1433 _ _ _ _]
          tunnel: w1429 -> [w1432 w1435 w1437 w1443 w1449]
          tunnel: w1428 -> [_ _ _ w1441 w1446]
          tunnel: [w1433 UI_State."Waiting for Exit (Acq Stopped)" ("UI State") UI_State."Waiting for Stop (Acq Stopped)" ("UI State") UI_State."Idle" ("UI State") UI_State."Idle" ("UI State")] -> w1427
          tunnel: [w1432 w1435 w1437 w1442 w1447] -> w1426
          frame Default {
          }
          frame "Waiting for Exit", "Waiting for Exit (Acq Stopped)" {
          }
          frame "Waiting for Stop", "Waiting for Stop (Acq Stopped)" {
          }
          frame "Waiting for Exit (Log Stopped)" {
            # "If we are waiting to exit, and the logging has already stopped, then the \"Acquisition Stopped\" message indicates that it is time to exit."
            n410 = call-poly "Enqueue Message.vi"("Priority Message? (F)"=TRUE, "error in (no error)"=w1443, "Message"="Exit", "Message Queue"=w1441) -> ("error out"=w1442:errorcluster)  [unwired: 6 in, 1 out]
          }
          frame "Waiting for Stop (Log Stopped)" {
            # "If we are waiting to stop, and the logging has already stopped, then the \"Acquisition Stopped\" message indicates that it is time to stop."
            n411 = call-poly "Enqueue Message.vi"("error in (no error)"=w1449, "Message Data"="Ready..." ("Ready..."), "Message"="Update Status", "Message Queue"=w1446) -> ("error out"=w1447:errorcluster)  [unwired: 6 in, 1 out]
          }
        }
      }
      frame "Logging Stopped" {
        # "Logic for determining what action to take when the logging has stopped."
        n412 = case shown="\"Waiting for Exit (Acq Stopped)\"" w1467 {
          selector: w1467 -> [w1469 _ _ _ _]
          tunnel: w1466 -> [w1468 w1471 w1473 w1479 w1482]
          tunnel: w1465 -> [_ _ _ w1477 w1481]
          tunnel: [w1469 UI_State."Waiting for Exit (Log Stopped)" ("UI State") UI_State."Waiting for Stop (Log Stopped)" ("UI State") UI_State."Idle" ("UI State") UI_State."Idle" ("UI State")] -> w1464
          tunnel: [w1468 w1471 w1473 w1478 w1480] -> w1463
          frame Default {
          }
          frame "Waiting for Exit", "Waiting for Exit (Log Stopped)" {
          }
          frame "Waiting for Stop", "Waiting for Stop (Log Stopped)" {
          }
          frame "Waiting for Exit (Acq Stopped)" {
            # "If we are waiting to exit, and the acquisition has already stopped, then the \"Logging Stopped\" message indicates that it is time to exit."
            n413 = call-poly "Enqueue Message.vi"("Priority Message? (F)"=TRUE, "error in (no error)"=w1479, "Message"="Exit", "Message Queue"=w1477) -> ("error out"=w1478:errorcluster)  [unwired: 6 in, 1 out]
          }
          frame "Waiting for Stop (Acq Stopped)" {
            # "If we are waiting to stop, and the acquisition has already stopped, then the \"Logging Stopped\" message indicates that it is time to stop."
            n414 = call-poly "Enqueue Message.vi"("error in (no error)"=w1482, "Message Data"="Ready..." ("Ready..."), "Message"="Update Status", "Message Queue"=w1481) -> ("error out"=w1480:errorcluster)  [unwired: 6 in, 1 out]
          }
        }
        n415 = Unbundle By Name(w1457) -> ("Exit Ref"=w1456:refnum<vi>, "Settings Ref"=w1455:refnum<vi>, "Start Ref"=w1454:refnum<vi>, "Stop Ref"=w1451:refnum<vi>)
        n416 = Build Array(w1456, w1455, w1454) -> (w1453:refnum<vi>[])
        n417 = call "Set Enable State on Multiple Controls.vi"("Enable?"=TRUE, "Controls"=w1453) -> ()  [unwired: 10 in]
        n418 = property class="Bool"(reference=w1451, "DisabledEnum"=T10."Disabled and Grayed Out" ("Disabled")) -> ()  [unwired: 1 in, 2 out]
      }
      frame "Launch Settings Dialog" {
        # "Launch Settings Dialog - Launch the Settings Dialog when the user clicks the 'Settings' button."
        n419 = call-by-ref "?"("error in (no error)"=w1498, "Settings in"=w1488) -> ("error out"=w1495:errorcluster, "Cancelled?"=w1497:bool, "Settings out"=w1491:T8)  [unwired: 8 in, 3 out]
        n420 = case shown="True" w1497 {
          tunnel: w1496 -> [w1502 _]
          tunnel: w1495 -> [w1501 w1503]
          tunnel: [w1500 w1503] -> w1492
          frame False {
            n421 = call-poly "Enqueue Message.vi"("error in (no error)"=w1501, "Message"="Broadcast Settings", "Message Queue"=w1502) -> ("error out"=w1500:errorcluster)  [unwired: 7 in, 1 out]
          }
          frame True {
          }
        }
      }
      frame "Broadcast Settings" {
        w1515 = "Update Settings" ("Message")
        # "Broadcast settings - Send the 'Update Settings' message to the Logging and Acquisition message loops."
        n422 = local read "Select LCR"() -> (w1511:refnum<visa-resource-name>)
        n423 = local read "IDN"() -> (w1510:string)
        n424 = local read "BIN State Read"() -> (w1509:bool)
        n425 = local read "Comparator Mode"() -> (w1508:u16)
        n426 = Bundle By Name(cluster=w1506, "VISA resource name"=w1511, "Logging Configuration.String"=w1510, "BIN State"=w1509, "Comparator Mode"=w1508) -> (w1512:T8)
        n427 = call-poly "Enqueue Message.vi"("Message Data"=w1512, "Message"=w1515, "Message Queue"=w1518) -> ("error out"=w1514:errorcluster)  [unwired: 7 in, 1 out]
        n428 = call-poly "Enqueue Message.vi"("error in (no error)"=w1514, "Message Data"=w1512, "Message"=w1515, "Message Queue"=w1519) -> ("error out"=w1513:errorcluster)  [unwired: 6 in, 1 out]
        n429 = Merge Errors(w1513, w1521) -> (w1522:errorcluster)
      }
      frame "Error" {
        # "Error - Display an error dialog. This message is sent by the \"Error Handler\" VIs at the end of other loops in this application."
        n430 = Variant To Data(error in=w1529, type=errorcluster {"status"=FALSE, "code"=0, "source"=""} ("error constant"), Variant=w1532) -> (data=w1530:errorcluster, error out=w1527:errorcluster)
        n431 = call <vilib>:"Simple Error Handler.vi"("error in (no error)"=w1530) -> ()  [unwired: 4 in, 5 out]
      }
      frame "Confirm Quit" {
        # "Confirm Quit - Message that can confirm whether or not the user wants to exit the application."
        n432 = case shown="\"Acquiring and Logging\"" w1544 {
          tunnel: w1543 -> [w1551 w1555]
          tunnel: w1542 -> [w1550 w1554]
          tunnel: [w1549 w1553] -> w1541
          tunnel: [UI_State."Idle" ("UI State") w1552] -> w1540
          frame Default {
            # "If 'Confirm Quit' comes in while the system is idle, there is no need for a confirmation message."
            n433 = call-poly "Enqueue Message.vi"("Priority Message? (F)"=TRUE, "error in (no error)"=w1550, "Message"="Exit", "Message Queue"=w1551) -> ("error out"=w1549:errorcluster)  [unwired: 6 in, 1 out]
          }
          frame "Acquiring and Logging" {
            n434 = Two Button Dialog(message="Are you sure you want to quit while the acquisition is running?" ("Confirm Quit Message"), 1:"No" ("No"), 2:"Yes" ("Yes")) -> (T button?=w1556:bool)
            n435 = case shown="False" w1556 {
              tunnel: w1555 -> [_ w1565]
              tunnel: w1554 -> [w1561 w1566]
              tunnel: [w1561 w1564] -> w1553
              tunnel: [UI_State."Acquiring and Logging" ("UI State") UI_State."Waiting for Exit" ("UI State")] -> w1552
              frame False {
                # "User did not want to quit."
              }
              frame True {
                n436 = call-poly "Enqueue Message.vi"("error in (no error)"=w1566, "Message"="Stop", "Message Queue"=w1565) -> ("error out"=w1564:errorcluster)  [unwired: 7 in, 1 out]
              }
            }
          }
        }
      }
      frame "Stop Acquisition" {
        w1569 = TRUE  # Priority Message
        w1577 = "Stop" ("Message")
        n437 = call-poly "Enqueue Message.vi"("Priority Message? (F)"=w1569, "error in (no error)"=w1570, "Message"=w1577, "Message Queue"=w1576) -> ("error out"=w1578:errorcluster)  [unwired: 6 in, 1 out]
        n438 = call-poly "Enqueue Message.vi"("Priority Message? (F)"=w1569, "error in (no error)"=w1578, "Message"=w1577, "Message Queue"=w1581) -> ("error out"=w1572:errorcluster)  [unwired: 6 in, 1 out]
        n439 = call-poly "Enqueue Message.vi"("Priority Message? (F)"=w1569, "error in (no error)"=w1572, "Message"="Exit", "Message Queue"=w1579) -> ("error out"=w1571:errorcluster)  [unwired: 6 in, 1 out]
      }
      frame "Disconnect" {
        w1600 = "stop" ("Message")
        # "Exit Acquisition and Logging loops, remains in the  Event Handling Loop."
        n440 = Variant To Data(type=errorcluster {"status"=FALSE, "code"=0, "source"=""} ("error constant"), Variant=w1602) -> (data=w1601:errorcluster)  [unwired: 1 in, 1 out]
        n441 = call <vilib>:"Simple Error Handler.vi"("error in (no error)"=w1601) -> ()  [unwired: 4 in, 5 out]
        n442 = call-poly "Enqueue Message.vi"("Priority Message? (F)"=TRUE, "error in (no error)"=w1597, "Message"=w1600, "Message Queue"=w1585) -> ("error out"=w1596:errorcluster)  [unwired: 6 in, 1 out]
        n443 = Flush Queue(queue=w1585, error in (no error)=w1597) -> (error out=w1595:errorcluster)  [unwired: 2 out]
        n444 = property on="Connect" class="Bool (strict)"("DisabledEnum"=T10."Enabled" ("Disabled")) -> ()  [unwired: 2 in, 2 out]
        n445 = local read "Start"() -> (w1587:bool)
        n446 = case shown="True" w1587 {
          tunnel: w1600 -> [_ w1613]
          tunnel: w1586 -> [_ w1612]
          tunnel: w1596 -> [w1606 w1611]
          tunnel: w1595 -> [w1607 w1610]
          tunnel: [w1607 w1609] -> w1593
          tunnel: [w1606 w1608] -> w1589
          frame False {
          }
          frame True {
            n447 = call-poly "Enqueue Message.vi"("error in (no error)"=w1611, "Message"=w1613, "Message Queue"=w1612) -> ("error out"=w1608:errorcluster)  [unwired: 7 in, 1 out]
            n448 = Flush Queue(queue=w1612, error in (no error)=w1610) -> (error out=w1609:errorcluster)  [unwired: 2 out]
          }
        }
        n449 = Merge Errors(w1589, w1593) -> (w1594:errorcluster)
      }
      frame "Exit" {
        w1629 = TRUE ("Priority Message? (F)")
        w1630 = "Exit" ("Message")
        # "Popup an error dialog if 'Exit' was called as a result of an error."
        # "Stop the VI"
        # "Exit - Send Exit messages to the Acquisition and Logging loops, and fire the user event to stop the Event Handling Loop."
        n450 = Variant To Data(type=errorcluster {"status"=FALSE, "code"=0, "source"=""} ("error constant"), Variant=w1632) -> (data=w1631:errorcluster)  [unwired: 1 in, 1 out]
        n451 = call <vilib>:"Simple Error Handler.vi"("error in (no error)"=w1631) -> ()  [unwired: 4 in, 5 out]
        n452 = call-poly "Enqueue Message.vi"("Priority Message? (F)"=w1629, "error in (no error)"=w1623, "Message"=w1630, "Message Queue"=w1625) -> ("error out"=w1622:errorcluster)  [unwired: 6 in, 1 out]
        n453 = Flush Queue(queue=w1625, error in (no error)=w1623) -> (error out=w1621:errorcluster)  [unwired: 2 out]
        n454 = call-poly "Enqueue Message.vi"("Priority Message? (F)"=w1629, "error in (no error)"=w1622, "Message"=w1630, "Message Queue"=w1624) -> ("error out"=w1617:errorcluster)  [unwired: 6 in, 1 out]
        n455 = Flush Queue(queue=w1624, error in (no error)=w1621) -> (error out=w1618:errorcluster)  [unwired: 2 out]
        n456 = call "Fire User Event - Stop.vi"("error in (no error)"=w1617, "User Event - Stop"=w1628) -> ("error out"=w1619:errorcluster)  [unwired: 9 in]
        n457 = Merge Errors(w1619, w1618) -> (w1620:errorcluster)
      }
      frame "---Copy This Frame---" {
        # "Duplicate this frame when creating new messages.  Change this comment in the duplicated frame to describe this message."
        n458 = Unbundle By Name(w1639) -> ()  [unwired: 1 out]
      }
      frame Default {
        # "'Default' case only runs if there is a message that isn't defined in any of the other cases.  Output a programming error."
        n459 = xnode "Error Ring"("parameter 0"=w1651) -> ("error out"=w1650:errorcluster)
      }
    }
    n460 = call "Error Handler - Message Handling Loop.vi"("error in (no error)"=w286, "Message Queue"=w273) -> ("dup error in"=w287:errorcluster)  [unwired: 8 in, 1 out]
  }
  n461 = while {
    tunnel: w25 -> [w1666]
    tunnel: [w1663] -> w35
    shift-right: [w1665] -> w31
    shift-left: w23 -> [w1667]
    stop <- w1664 stop-if-true
    # "Event Handling Loop"
    n462 = event shown="[25] \"Tab Control\": Value Change" {
      selector: w1667 -> [_ _ _ _ _ _ _ _ _ _ _ _ _ _ _ _ _ _ _ _ _ _ _ _ _ _ _ _ _ _ _ _ _]
      dyn-events: [_ _ _ _ _ _ _ _ _ _ _ _ _ _ _ _ _ _ _ _ _ _ _ _ _ _ _ _ _ _ _ _ _] -> w1665
      timeout: _ -> [_ _ _ _ _ _ _ _ _ _ _ _ _ _ _ _ _ _ _ _ _ _ _ _ _ _ _ _ _ _ _ _ _]
      tunnel: [_ _ _ _ _ _ _ _ _ _ _ _ _ _ _ _ _ _ _ _ _ _ _ _ _ _ _ _ _ _ _ _ TRUE ("Discard?")] -> w1664
      tunnel: w1666 -> [w1668 w1674 w1678 w1683 w1686 w1690 w1695 w1698 w1702 w1704 w1709 w1713 w1716 w1719 w1722 w1725 w1729 w1735 w1741 w1747 w1752 w1756 w1760 w1764 w1768 w1773 w1777 w1780 w1784 w1788 w1791 w1794 w1798]
      tunnel: [w1670 w1672 w1676 w1680 w1684 w1687 w1692 _ w1699 _ w1706 w1711 _ _ _ _ w1727 w1733 w1740 w1746 _ w1753 w1759 w1762 w1766 _ w1775 w1779 _ w1786 _ w1797 _] -> w1662
      tunnel: [w1669 w1673 w1677 w1682 w1686 w1689 w1694 w1697 w1701 w1703 w1707 w1712 w1715 w1718 w1721 w1724 w1726 w1734 w1736 w1742 w1751 w1755 w1757 w1763 w1767 w1772 w1776 w1778 w1783 w1787 w1791 w1793 w1798] -> w1661
      event "Start": Value Change {
        n463 = event-data() -> ()  [unwired: 1 in, 1 out]
        n464 = call-poly "Enqueue Message.vi"("Message"="Start", "Message Queue"=w1668) -> ("error out"=w1670:errorcluster, "dup Message Queue"=w1669:refnum<queue>)  [unwired: 8 in]
      }
      event "Connect": Value Change {
        n465 = event-data() -> ()  [unwired: 1 in, 1 out]
        n466 = call-poly "Enqueue Message.vi"("Message"="Initialize Instrument", "Message Queue"=w1674) -> ("error out"=w1672:errorcluster, "dup Message Queue"=w1673:refnum<queue>)  [unwired: 8 in]
      }
      event "Settings": Value Change {
        n467 = event-data() -> ()  [unwired: 1 in, 1 out]
        n468 = call-poly "Enqueue Message.vi"("Message"="Launch Settings Dialog", "Message Queue"=w1678) -> ("error out"=w1676:errorcluster, "dup Message Queue"=w1677:refnum<queue>)  [unwired: 8 in]
      }
      event "Speed", "Function", "Range": Value Change {
        n469 = event-data() -> ()  [unwired: 1 in, 6 out]
        n470 = call-poly "Enqueue Message.vi"("Message"="Measurement Config", "Message Queue"=w1683) -> ("error out"=w1680:errorcluster, "dup Message Queue"=w1682:refnum<queue>)  [unwired: 8 in]
      }
      event "Frequency", "Level": Value Change; "Level": event #0x43; "Level": Operate Menu Activation {
        n471 = event-data() -> ()  [unwired: 1 in, 1 out]
        n472 = call-poly "Enqueue Message.vi"("Message"="MEAS SIGNAL", "Message Queue"=w1686) -> ("error out"=w1684:errorcluster)  [unwired: 8 in, 1 out]
      }
      event "Count State": Value Change {
        n473 = event-data() -> ()  [unwired: 1 in, 1 out]
        n474 = call-poly "Enqueue Message.vi"("Message"="BIN Count", "Message Queue"=w1690) -> ("error out"=w1687:errorcluster, "dup Message Queue"=w1689:refnum<queue>)  [unwired: 8 in]
      }
      event "Enable Sweep": Value Change {
        n475 = event-data() -> ("NewVal"=→"Enable Sweep New Value":bool)  [unwired: 1 in, 1 out]
        n476 = call-poly "Enqueue Message.vi"("Message"="Enable Sweep", "Message Queue"=w1695) -> ("error out"=w1692:errorcluster, "dup Message Queue"=w1694:refnum<queue>)  [unwired: 8 in]
      }
      event "Sweep Function": Value Change {
        n477 = event-data() -> ()  [unwired: 1 in, 1 out]
        n478 = call-poly "Enqueue Message.vi"("Message"="Sweep Function", "Message Queue"=w1698) -> ("dup Message Queue"=w1697:refnum<queue>)  [unwired: 8 in, 1 out]
      }
      event "Sweep Mode": Value Change {
        n479 = event-data() -> ()  [unwired: 1 in, 1 out]
        n480 = call-poly "Enqueue Message.vi"("Message"="Sweep Mode", "Message Queue"=w1702) -> ("error out"=w1699:errorcluster, "dup Message Queue"=w1701:refnum<queue>)  [unwired: 8 in]
      }
      event "Sweep Parameter": Value Change {
        n481 = event-data() -> ()  [unwired: 1 in, 1 out]
        n482 = call-poly "Enqueue Message.vi"("Message"="Sweep Swap", "Message Queue"=w1704) -> ("dup Message Queue"=w1703:refnum<queue>)  [unwired: 8 in, 1 out]
      }
      event "Interpolation": Value Change {
        n483 = event-data() -> ()  [unwired: 1 in, 1 out]
        n484 = call-poly "Enqueue Message.vi"("Message"="Sweep Interpolation", "Message Queue"=w1709) -> ("error out"=w1706:errorcluster, "dup Message Queue"=w1707:refnum<queue>)  [unwired: 8 in]
      }
      event "Sweep Points": Value Change {
        n485 = event-data() -> ()  [unwired: 1 in, 1 out]
        n486 = call-poly "Enqueue Message.vi"("Message"="Sweep Step", "Message Queue"=w1713) -> ("error out"=w1711:errorcluster, "dup Message Queue"=w1712:refnum<queue>)  [unwired: 8 in]
      }
      event "Autoscale Frequency": Value Change {
        n487 = event-data() -> ()  [unwired: 1 in, 1 out]
        n488 = call-poly "Enqueue Message.vi"("Message"="Sweep Frequency Autoscale", "Message Queue"=w1716) -> ("dup Message Queue"=w1715:refnum<queue>)  [unwired: 8 in, 1 out]
      }
      event "Start Frequency", "Stop Frequency": Value Change {
        n489 = event-data() -> ()  [unwired: 1 in, 1 out]
        n490 = call-poly "Enqueue Message.vi"("Message"="Sweep Range", "Message Queue"=w1719) -> ("dup Message Queue"=w1718:refnum<queue>)  [unwired: 8 in, 1 out]
      }
      event "Autoscale Limit": Value Change {
        n491 = event-data() -> ()  [unwired: 1 in, 1 out]
        n492 = call-poly "Enqueue Message.vi"("Message"="Sweep Limit Autoscale", "Message Queue"=w1722) -> ("dup Message Queue"=w1721:refnum<queue>)  [unwired: 8 in, 1 out]
      }
      event "Sweep Low Limit", "Sweep High Limit": Value Change {
        n493 = event-data() -> ()  [unwired: 1 in, 1 out]
        n494 = call-poly "Enqueue Message.vi"("Message"="Sweep Limit Range", "Message Queue"=w1725) -> ("dup Message Queue"=w1724:refnum<queue>)  [unwired: 8 in, 1 out]
      }
      event "Trigger": Value Change {
        n495 = event-data() -> ()  [unwired: 1 in, 1 out]
        n496 = call-poly "Enqueue Message.vi"("Message"="Trigger BIN", "Message Queue"=w1729) -> ("error out"=w1727:errorcluster, "dup Message Queue"=w1726:refnum<queue>)  [unwired: 8 in]
      }
      event "BIN No..BIN 1", "BIN No..BIN 2", "BIN No..BIN 3", "BIN No..BIN 4", "BIN No..BIN 5", "BIN No..BIN 6", "BIN No..BIN 7", "BIN No..BIN 8", "BIN No..BIN 9", "BIN No..SEC": Value Change {
        n497 = event-data() -> ("CtlRef"=→"BIN REF":refnum<vi>, "NewVal"=→"New BIN State":bool)  [unwired: 1 in, 4 out]
        n498 = call-poly "Enqueue Message.vi"("Message"="Set BIN State", "Message Queue"=w1735) -> ("error out"=w1733:errorcluster, "dup Message Queue"=w1734:refnum<queue>)  [unwired: 8 in]
      }
      event "Low Limit.BIN 1", "Low Limit.BIN 2", "Low Limit.BIN 3", "Low Limit.BIN 4", "Low Limit.BIN 5", "Low Limit.BIN 6", "Low Limit.BIN 7", "Low Limit.BIN 8", "Low Limit.BIN 9", "Low Limit.SEC": Value Change {
        n499 = event-data() -> ("CtlRef"=→"Low Limit Ref":refnum<vi>, "NewVal"=→"New Low Limit Val":dbl)  [unwired: 1 in, 4 out]
        n500 = call-poly "Enqueue Message.vi"("Message"="BIN Low Limit", "Message Queue"=w1741) -> ("error out"=w1740:errorcluster, "dup Message Queue"=w1736:refnum<queue>)  [unwired: 8 in]
      }
      event "High Limit.BIN 1", "High Limit.BIN 2", "High Limit.BIN 3", "High Limit.BIN 4", "High Limit.BIN 5", "High Limit.BIN 6", "High Limit.BIN 7", "High Limit.BIN 8", "High Limit.BIN 9", "High Limit.SEC": Value Change {
        n501 = event-data() -> ("CtlRef"=→"High Limit Ref":refnum<vi>, "NewVal"=→"New High Limit Val":dbl)  [unwired: 1 in, 4 out]
        n502 = call-poly "Enqueue Message.vi"("Message"="BIN High Limit", "Message Queue"=w1747) -> ("error out"=w1746:errorcluster, "dup Message Queue"=w1742:refnum<queue>)  [unwired: 8 in]
      }
      event "Nominal Value (0.0)": Value Change {
        n503 = event-data() -> ("CtlRef"=→"CtlRef":refnum<vi>, "OldVal"=→"OldVal":dbl)  [unwired: 1 in, 4 out]
        n504 = call-poly "Enqueue Message.vi"("Message"="BIN Nominal", "Message Queue"=w1752) -> ("dup Message Queue"=w1751:refnum<queue>)  [unwired: 8 in, 1 out]
      }
      event "Sweep Display Mode": Value Change {
        n505 = event-data() -> ()  [unwired: 1 in, 6 out]
        n506 = call-poly "Enqueue Message.vi"("Message"="Sweep Display Mode", "Message Queue"=w1756) -> ("error out"=w1753:errorcluster, "dup Message Queue"=w1755:refnum<queue>)  [unwired: 8 in]
      }
      event "Comparator Swap": Value Change {
        n507 = event-data() -> ()  [unwired: 1 in, 1 out]
        n508 = call-poly "Enqueue Message.vi"("Message"="Comparator  Swap", "Message Queue"=w1760) -> ("error out"=w1759:errorcluster, "dup Message Queue"=w1757:refnum<queue>)  [unwired: 8 in]
      }
      event "Comparator Mode", "Bin Display Mode": Value Change {
        n509 = event-data() -> ()  [unwired: 1 in, 6 out]
        n510 = call-poly "Enqueue Message.vi"("Message"="BIN Config", "Message Queue"=w1764) -> ("error out"=w1762:errorcluster, "dup Message Queue"=w1763:refnum<queue>)  [unwired: 8 in]
      }
      event "Clear Count": Value Change {
        n511 = event-data() -> ()  [unwired: 1 in, 1 out]
        n512 = call-poly "Enqueue Message.vi"("Message"="BIN Clear", "Message Queue"=w1768) -> ("error out"=w1766:errorcluster, "dup Message Queue"=w1767:refnum<queue>)  [unwired: 8 in]
      }
      event "Tab Control": Value Change {
        n513 = event-data() -> ("CtlRef"=→"Tab Ref":refnum<vi>, "NewVal"=→"NewVal":enum32{"BIN", "SWEEP"})  [unwired: 1 in, 4 out]
        n514 = call-poly "Enqueue Message.vi"("Message"="Tab Control", "Message Queue"=w1773) -> ("dup Message Queue"=w1772:refnum<queue>)  [unwired: 8 in, 1 out]
      }
      event "Beeper Mode": Value Change; "Beeper Mode": Operate Menu Activation {
        n515 = event-data() -> ()  [unwired: 1 in, 1 out]
        n516 = call-poly "Enqueue Message.vi"("Message"="Beeper Mode", "Message Queue"=w1777) -> ("error out"=w1775:errorcluster, "dup Message Queue"=w1776:refnum<queue>)  [unwired: 8 in]
      }
      event "Stop": Value Change {
        n517 = event-data() -> ()  [unwired: 1 in, 1 out]
        n518 = call-poly "Enqueue Message.vi"("Message"="Stop", "Message Queue"=w1780) -> ("error out"=w1779:errorcluster, "dup Message Queue"=w1778:refnum<queue>)  [unwired: 8 in]
      }
      event "Disconnect": Value Change {
        n519 = event-data() -> ()  [unwired: 1 in, 1 out]
        n520 = call-poly "Enqueue Message.vi"("Message"="Disconnect", "Message Queue"=w1784) -> ("dup Message Queue"=w1783:refnum<queue>)  [unwired: 8 in, 1 out]
      }
      event Panel Close? {
        # "Send the 'Confirm Quit' message if the user closes the panel of the VI. Discard the event so the 'Confirm Quit' message has a chance to run."
        n521 = event-data() -> ()  [unwired: 1 in, 1 out]
        n522 = call-poly "Enqueue Message.vi"("Priority Message? (F)"=TRUE, "Message"="Confirm Quit", "Message Queue"=w1788) -> ("error out"=w1786:errorcluster, "dup Message Queue"=w1787:refnum<queue>)  [unwired: 7 in]
        n523 = event-data("Discard?"=TRUE) -> ()  [unwired: 1 in, 1 out]
      }
      event Application Instance Close {
        n524 = event-data() -> ()  [unwired: 1 in, 1 out]
      }
      event "Disconnect": Value Change {
        w1795 = TRUE  # Priority Message
        n525 = event-data() -> ()  [unwired: 1 in, 1 out]
        n526 = property on="Connect" class="Bool (strict)"("DisabledEnum"=T10."Enabled" ("Disabled")) -> ()  [unwired: 2 in, 2 out]
        n527 = call-poly "Enqueue Message.vi"("Priority Message? (F)"=w1795, "Message"="Stop Acquisition", "Message Queue"=w1794) -> ("error out"=w1797:errorcluster, "dup Message Queue"=w1793:refnum<queue>)  [unwired: 7 in]
      }
      event User Event {
        # "The Message Handling Loop processed an \"Exit\" message, which fired this event to stop the Event Handling Loop."
        n528 = event-data() -> ()  [unwired: 1 in, 1 out]
        n529 = local write "Status"("Exit" ("Exit String")) -> ()
      }
    }
    n530 = call "Error Handler - Event Handling Loop.vi"("error in (no error)"=w1662, "Message Queue"=w1661) -> ("dup error in"=w1663:errorcluster)  [unwired: 8 in, 1 out]
  }
  n531 = Obtain Notifier(notification data type="BIN Read In") -> (notifier out=w12:refnum<notifier>)  [unwired: 3 in, 2 out]
  n532 = call "Acquisition Message Loop.vi"("BIN Notifier"=w12, "error in (no error)"=w15, "Data Notifier"=w5, "Data Queue"=w10, "Message Queues"=w9) -> ("error out"=w34:errorcluster)  [unwired: 6 in]
  n533 = while "Data Display Loop" {
    tunnel: w12 -> [w1806]
    stop <- w1807 stop-if-true
    # "BIN Data Display Loop"
    n534 = Wait on Notification(notifier=w1806) -> (notification=w1805:T1, error out=w1807:errorcluster)  [unwired: 3 in, 2 out]
    n535 = Unbundle By Name(w1805) -> ("Low Limit Read"=→"Low Limit Read":dbl[], "High Limit Read"=→"High Limit Read":dbl[], "BIN Count Array"=→"BIN Result":i32[], "Nominal"=→"Nominal":string)
  }
  n536 = Release Queue(queue=w25, error in (no error)=w36) -> (error out=w8:errorcluster)  [unwired: 1 in, 2 out]
  n537 = Unregister For Events(event registration refnum=w31, error in=w35) -> (error out=w19:errorcluster)
  n538 = Release Notifier(notifier=w12, error in (no error)=w8) -> (error out=w7:errorcluster)  [unwired: 1 in, 2 out]
  n539 = Release Notifier(notifier=w5, error in (no error)=w7) -> (error out=w6:errorcluster)  [unwired: 1 in, 2 out]
  n540 = Release Queue(queue=w10, error in (no error)=w6) -> (error out=w11:errorcluster)  [unwired: 1 in, 2 out]
  n541 = Merge Errors(w19, w11, w34, w32) -> (w26:errorcluster)
  n542 = call "Destroy User Event - Stop.vi"("error in (no error)"=w26, "User Event - Stop"=w4) -> ("error out"=w24:errorcluster)  [unwired: 9 in]
  n543 = disable-structure shown="Default" {
    disable-tunnel: w24 -> [_ _]
    frame condition #0 (active) {
    }
    frame condition #1 {
      # "Call Quit LabVIEW if running as a built application."
      n544 = Quit LabVIEW() -> ()  [unwired: 1 in]
    }
  }
  "Color Box" <- u32 11347 ("Color Box")
